vi "DAQ_Main.vi"() -> ()   [LabVIEW 2016]
doc: "Main vi to collect ams data with the pixie 4."
uses:
  spectrum/controls/count control.ctl
  stable current/stable controls/stable cluster.ctl
  record data/realtime data/pixie vis/controls/measurement values.ctl
  record data/realtime data/pixie vis/controls/sample info cluster.ctl
  controls/rare event data.ctl
  controls/stable data.ctl
  controls/main state control.ctl
  controls/SCA broadcast status.ctl
  controls/read write shift control.ctl
  controls/SCA commands.ctl
  <vilib>/addons/database/Connection.llb/DB Tools Open Connec (String).vi
  <vilib>/addons/database/Connection.llb/Conn Execute.vi
  <vilib>/addons/database/Recordset.llb/Rec Fetch Recordset Data (R).vi
  <vilib>/addons/database/Recordset.llb/Rec Destroy - Connection.vi
  <vilib>/Utility/file.llb/Read Delimited Spreadsheet (DBL).vi
  <vilib>/addons/database/NI_Database_API.lvlib
panel:
  out "SCA status":T1
  out "DAQ state control":T2
  in  "Stable Data":T3
  in  "Rare Event Data":T4
  in  "skip sample":bool
  out "Measurement values 3":T5={"Cycle number"=2461.0, "Transmission"=28.91860852171752, "Current 1"=9198.03481365116, " run time"=7.303, "Counts"=606.0, "Live Time"=0.9930715935334873, "Counts per minute"=5013.511490976947, "2nd Current 1"=9198.03481365116, "10Be vs O17"=11.632407319707596, "O17 cycle Error"=52.09583737437704, "rare/stable"=4366.328416433736, "Cycle Error"=1.0, "Interference rate(cps"=144.89870339129973, "total interference counts"=1136.0, "SS Injector "=3.1190766269837584, "SS High End"=2.886696509772986} {"10Be vs O17" format="%#_6f"; "rare/stable" format="%#_6f"}
  in  "use SS ratio":u16(ring) items=["other", "36Cl"]
  out "change sample":i16
  in  "sample change failure":u32(colorbox)
  out "Sample DB fetch error":errorcluster
  in  "2nd sample warm up time 2":dbl=60.0
  in  "Wheel Name":string="tune 1"
  in  "run number":string="201502"
  in  "wheelnumber":string="1"
  in  "runletter":string="2015_14C-01"
  out "run time(sec)":dbl=7.303 format="%#_4g"
  out "sample warm up":u32=200
  in  "number of cycles":u32=4
  in  "1st sample warm up time":dbl=200.0
  in  "run time":dbl=60.0
  out "first time run":bool
  out "recordset data":variant[][](array[variant])
  out "Rare Event Window error":errorcluster
  out "DAQ running SV error":errorcluster
  out "Sample Change Start SV error":errorcluster
  out "input count rate 0":dbl=145.76259366407135
  out "run data output":T6={"input count rate 0"=145.76259366407135, "input count rate 1"=146.1439819888232, "input count rate 2"=0.0, "input count rate 3"=0.0, "number of events"=1136.0, "event rate"=144.89870339129973}
  in  "time for each measurement":i32=500
  in  "data out":T7={"Total counts"=4140, "cps"=80.49411774042008, "live time"=0.9916920520631404, "pulser"=3611.0, "rare counts"=4809.0, "other counts"=4294958918.0, "total run time(sec)"=60.244, "adjusted run time(sec)"=59.74349598449183, "17O average"=4.140581045750721, "17O current"=372.65229411756485}
  in  "abort count rate (cps)":dbl=40000.0
  in  "reset":bool
  out "rare count rate":dbl=54.0 format="%#_3g"
  out "DB input error":errorcluster
  in  "13 to 12 conversion .011 for 14C otherwise 1":dbl=1.0
  in  "Charge State":dbl=3.0
  out "Measurement values 2":T8={"Cycle number"=2461.0, "Transmission"=28.91860852171752, "Current 1"=9198.03481365116, " run time"=7.303, "Counts"=606.0, "Live Time"=0.9930715935334873, "Counts per minute"=5013.511490976947, "2nd Current 1"=9198.03481365116, "10Be vs O17"=11.632407319707596, "O17 cycle Error"=52.09583737437704, "rare/stable"=4366.328416433736, "Cycle Error"=1.0, "Interference rate(cps"=144.89870339129973, "total interference counts"=1136.0, "SS Injector "=3.1190766269837584, "SS High End"=2.886696509772986} {"10Be vs O17" format="%#_6f"; "rare/stable" format="%#_6f"}
  out "Sample information":T9={"Cathode Number"="124120", "Sample Name"="26Al-01-5-1", "Type"="s", "User Name"="Caffee", "Cycles Measured"="1", "Cathode Position"="10", "Estimated Ratio"="4694"}
  in  "Measurement values":T8={"Cycle number"=2460.0, "Transmission"=24.878524366136492, "Current 1"=7973.094300785374, " run time"=60.244, "Counts"=4809.0, "Live Time"=0.9916920520631404, "Counts per minute"=4829.647064425205, "2nd Current 1"=7951.125552694256, "10Be vs O17"=12.904791077128992, "O17 cycle Error"=372.65229411756485, "rare/stable"=4859.10919175385, "Cycle Error"=1.0, "Interference rate(cps"=140.58271554902092, "total interference counts"=8495.0, "SS Injector "=3.1190766269837584, "SS High End"=2.886696509772986} {"10Be vs O17" format="%#_6f"; "rare/stable" format="%#_6f"}
  out "millisecond timer value":u32
  out "Wheel run order array":string[][](array[string])=[["10", "124120", "Caffee", "26Al-01-5-1", "s", "4694", "0", "Finished"], ["13", "109265", "Caffee", "QA-Al-16760", "u", "16760", "0", ""], ["12", "124831", "Caffee", "QA-Al-10650", "u", "10650", "0", ""], ["11", "123809", "Caffee", "QA-Al-499", "u", "499", "0", ""], ["4", "124041", "Sharma", "Blank", "b", "5", "0", ""], ["9", "124119", "Caffee", "26Al-01-5-1", "s", "4694", "0", ""], ["3", "124039", "Sharma", "Blank", "b", "5", "0", ""], ["2", "124035", "Sharma", "Blank", "b", "5", "0", ""], ["1", "124031", "Sharma", "Blank", "b", "5", "0", ""], ["8", "124118", "Caffee", "26Al-01-5-1", "s", "4694", "0", ""], ["10", "124120", "Caffee", "26Al-01-5-1", "s", "4694", "0", ""], ["13", "109265", "Caffee", "QA-Al-16760", "u", "16760", "0", ""], ["12", "124831", "Caffee", "QA-Al-10650", "u", "10650", "0", ""], ["11", "123809", "Caffee", "QA-Al-499", "u", "499", "0", ""], ["4", "124041", "Sharma", "Blank", "b", "5", "0", ""], ["9", "124119", "Caffee", "26Al-01-5-1", "s", "4694", "0", ""], ["3", "124039", "Sharma", "Blank", "b", "5", "0", ""], ["2", "124035", "Sharma", "Blank", "b", "5", "0", ""], ["1", "124031", "Sharma", "Blank", "b", "5", "0", ""], ["8", "124118", "Caffee", "26Al-01-5-1", "s", "4694", "0", ""], ["10", "124120", "Caffee", "26Al-01-5-1", "s", "4694", "0", ""], ["13", "109265", "Caffee", "QA-Al-16760", "u", "16760", "0", ""], ["12", "124831", "Caffee", "QA-Al-10650", "u", "10650", "0", ""], ["11", "123809", "Caffee", "QA-Al-499", "u", "499", "0", ""], ["4", "124041", "Sharma", "Blank", "b", "5", "0", ""], ["9", "124119", "Caffee", "26Al-01-5-1", "s", "4694", "0", ""], ["3", "124039", "Sharma", "Blank", "b", "5", "0", ""], ["2", "124035", "Sharma", "Blank", "b", "5", "0", ""], ["1", "124031", "Sharma", "Blank", "b", "5", "0", ""], ["8", "124118", "Caffee", "26Al-01-5-1", "s", "4694", "0", ""]]
  out "sample number":u16=57
  in  "stable data out 2":T10={"injector current"=10618.359999999999, "offset current"=7973.094300785374, "ss inj ratio"=3.1190766269837584, "ss offset ratio"=2.886696509772986, "transmission"=25.029271001000076, "2nd offset current"=7951.125552694256}
  out "stable data out":T10={"injector current"=10602.21, "offset current"=9198.03481365116, "ss inj ratio"=3.1190766269837584, "ss offset ratio"=2.886696509772986, "transmission"=28.91860852171752, "2nd offset current"=9198.03481365116}
  out "data":T7={"Total counts"=962, "cps"=83.5585248496158, "live time"=0.9930715935334873, "pulser"=433.0, "rare counts"=606.0, "other counts"=4294966311.0, "total run time(sec)"=7.303, "adjusted run time(sec)"=7.252401847575058, "17O average"=4.735985215852458, "17O current"=52.09583737437704}
  out "Event structure error out":errorcluster
  in  "run":bool=TRUE
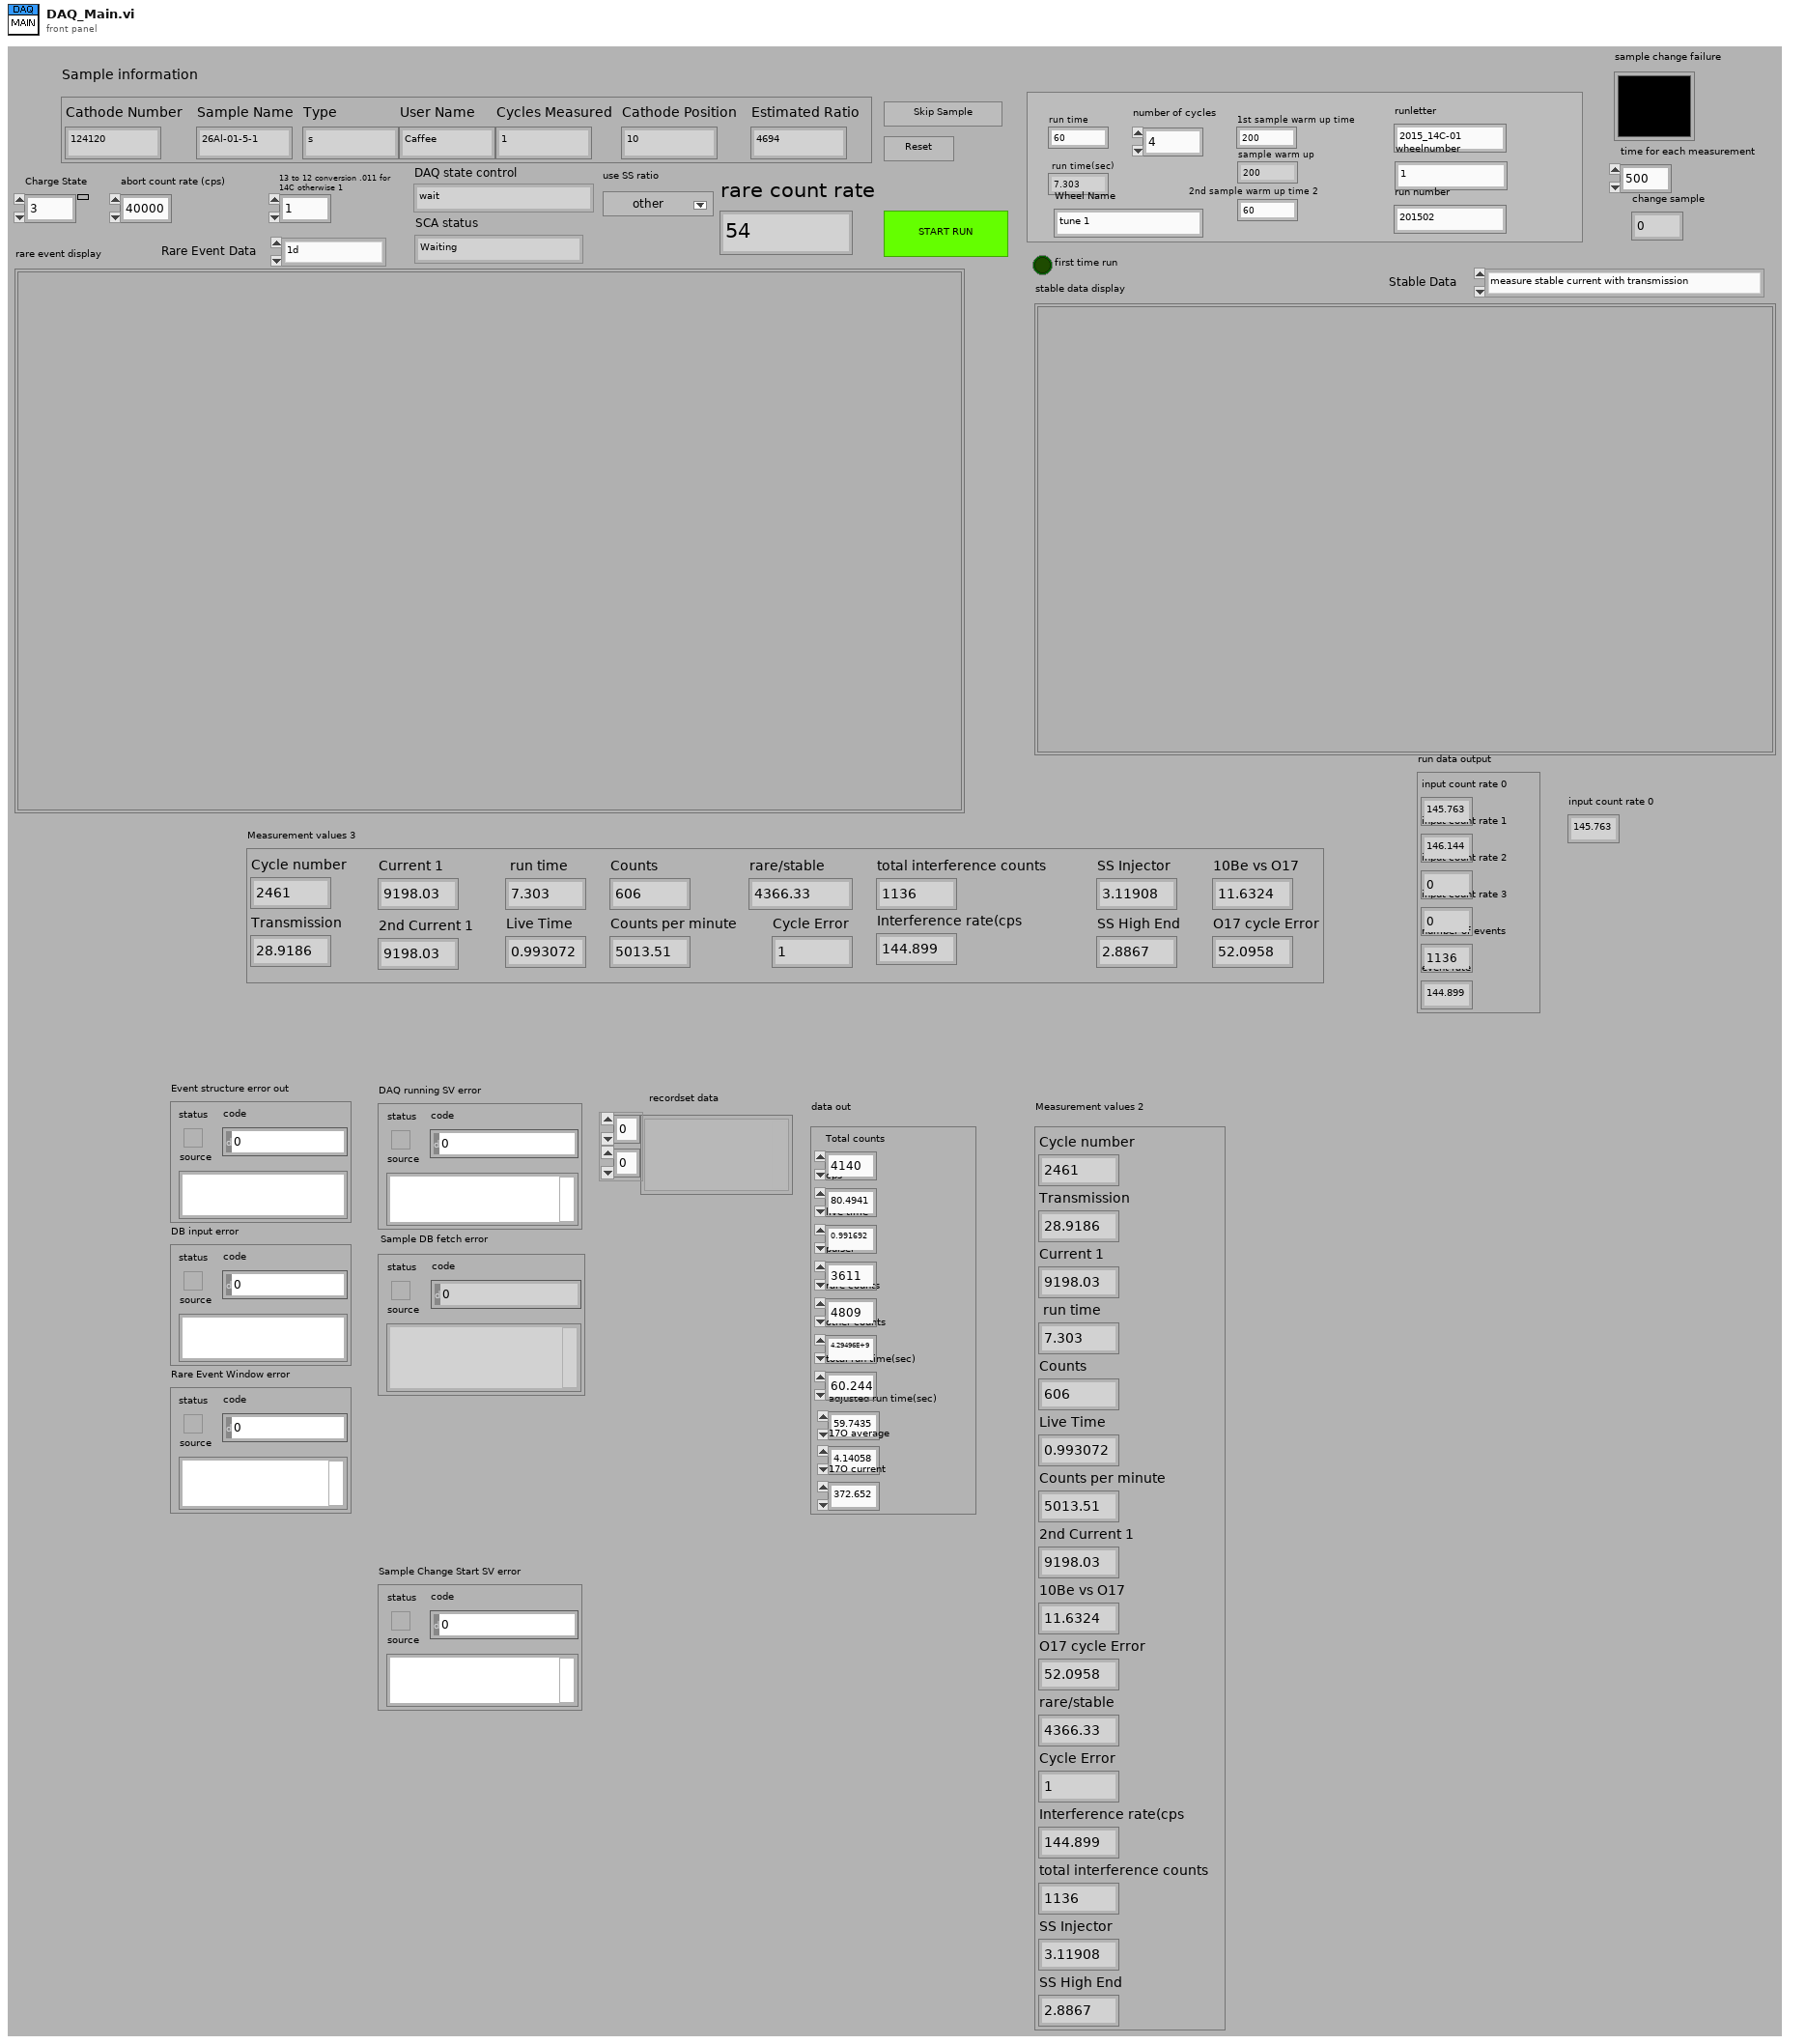
[diagram p1: front panel]
types:
  T1 = typedef "SCA broadcast status.ctl" = enum16{"Waiting", "Changing samples", "Sample change complete", "Failure"}
  T2 = typedef "main state control.ctl" = enum16{"wait", "set gate", "check injector cup", "start rare", "get rare", "stop rare", "abort run", "change sample", "wait for sample change", "check sample start", "insert cup", "remove cup", "sample warm up", "record data", "get transmission", "get stable"}
  T3 = typedef "stable data.ctl" = enum16{"measure stable current with transmission", "measure stable current", "35Cl + 37Cl measure stable current", "35Cl + 37Cl inj - 35Cl HE"}
  T4 = typedef "rare event data.ctl" = enum16{"1d", "2d", "2d 10Be"}
  T5 = cluster{"Cycle number":dbl, "Transmission":dbl, "Current 1":dbl, " run time":dbl, "Counts":dbl, "Live Time":dbl, "Counts per minute":dbl, "2nd Current 1":dbl, "10Be vs O17":dbl, "O17 cycle Error":dbl, "rare/stable":dbl, "Cycle Error":dbl, "Interference rate(cps":dbl, "total interference counts":dbl, "SS Injector ":dbl, "SS High End":dbl}
  T6 = cluster{"input count rate 0":dbl, "input count rate 1":dbl, "input count rate 2":dbl, "input count rate 3":dbl, "number of events":dbl, "event rate":dbl}
  T7 = typedef "count control.ctl" = cluster{"Total counts":u32, "cps":dbl, "live time":dbl, "pulser":dbl, "rare counts":dbl, "other counts":dbl, "total run time(sec)":dbl, "adjusted run time(sec)":dbl, "17O average":dbl, "17O current":dbl}
  T8 = typedef "measurement values.ctl" = cluster{"Cycle number":dbl, "Transmission":dbl, "Current 1":dbl, " run time":dbl, "Counts":dbl, "Live Time":dbl, "Counts per minute":dbl, "2nd Current 1":dbl, "10Be vs O17":dbl, "O17 cycle Error":dbl, "rare/stable":dbl, "Cycle Error":dbl, "Interference rate(cps":dbl, "total interference counts":dbl, "SS Injector ":dbl, "SS High End":dbl}
  T9 = typedef "sample info cluster.ctl" = cluster{"Cathode Number":string, "Sample Name":string, "Type":string, "User Name":string, "Cycles Measured":string, "Cathode Position":string, "Estimated Ratio":string}
  T10 = typedef "stable cluster.ctl" = cluster{"injector current":dbl, "offset current":dbl, "ss inj ratio":dbl, "ss offset ratio":dbl, "transmission":dbl, "2nd offset current":dbl}
  T11 = cluster{"array out[0]":string, "array out[1]":string, "array out[2]":string, "array out[3]":string, "array out[4]":string, "array out[5]":string, "array out[6]":string}
  T12 = typedef "read write shift control.ctl" = string
  T13 = typedef "SCA commands.ctl" = enum16{"Wait", "Shutdown", "Retract insert rod", "Insert insert rod", "Retract retract rod", "Insert retract rod", "Retract sample rod", "Insert sample rod", "Open wheel GV", "Close wheel GV", "Open ion source GV", "Close ion source GV", "Pump out source", "Vent source", "Rotate wheel randomly", "Rotate wheel", "Start random sample change", "Start sample change"}
  T14 = enum16{"open", "replace", "create", "open or create", "replace or create", "replace or create with confirmation"}
  T15 = typedef "NI_Database_API.lvlib/Conn ObjectReference.ctl" = refnum<k1>
  T16 = typedef "NI_Database_API.lvlib/Rec ObjectReference.ctl" = refnum<k1>
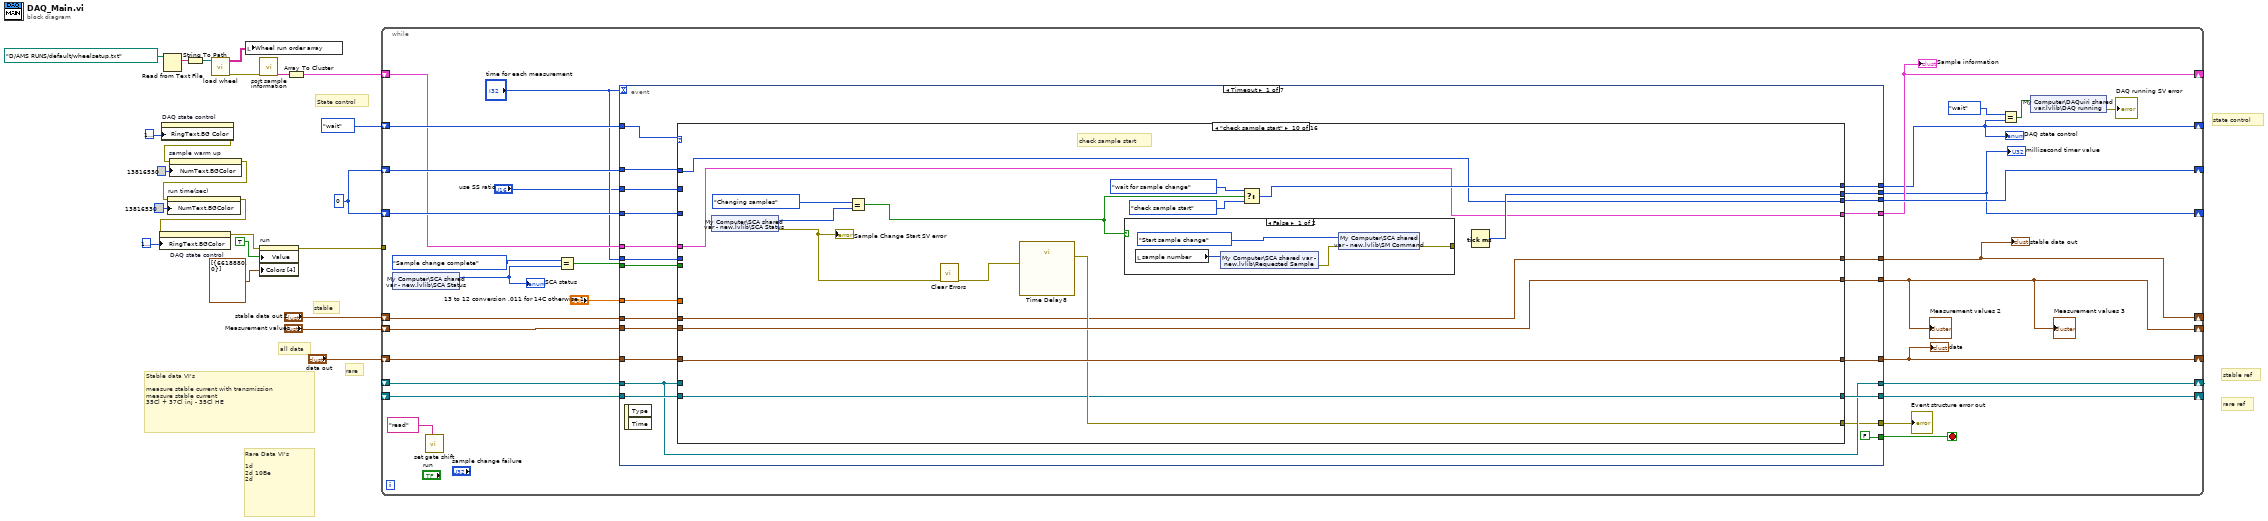
[diagram p0: block diagram]
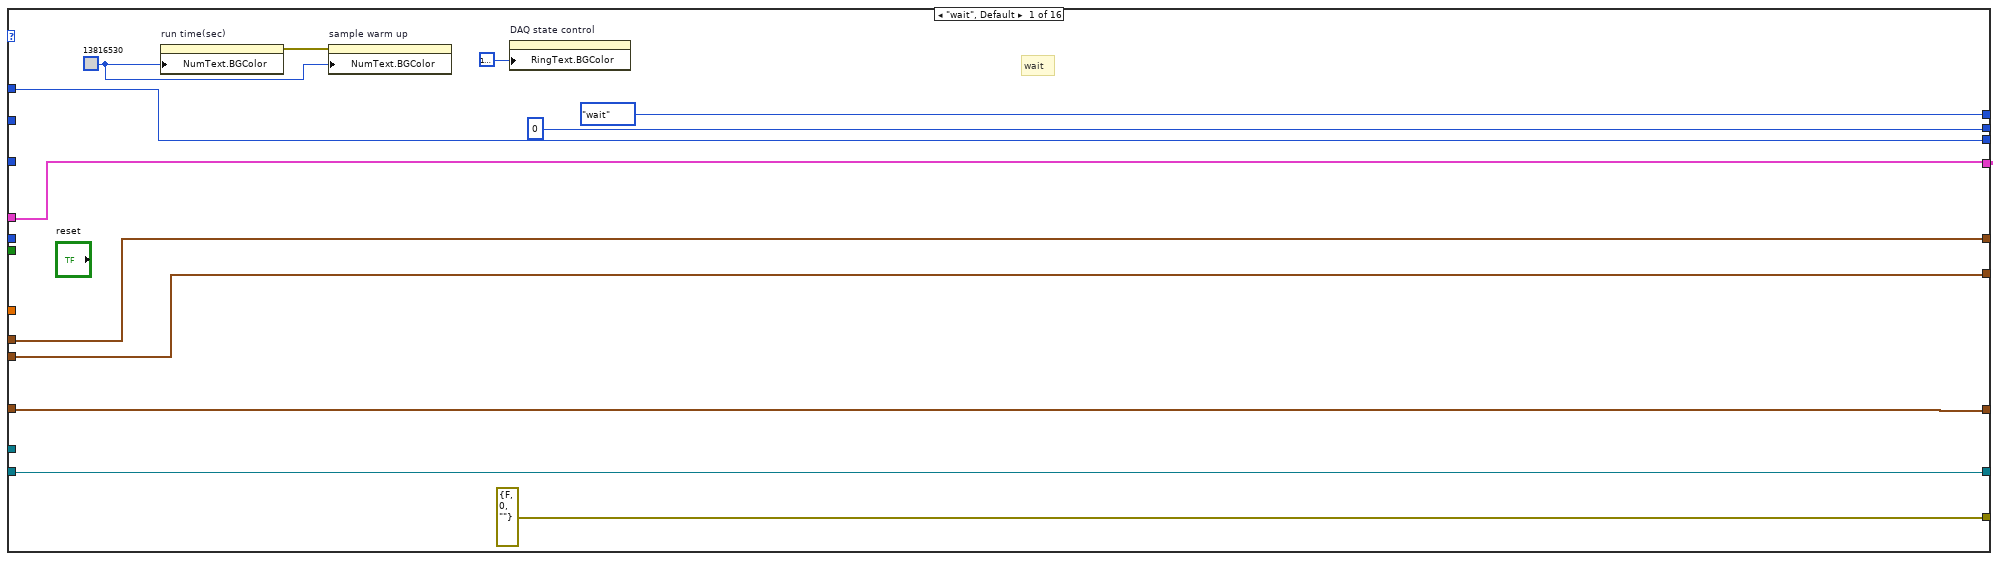
[diagram p2: hidden frame]
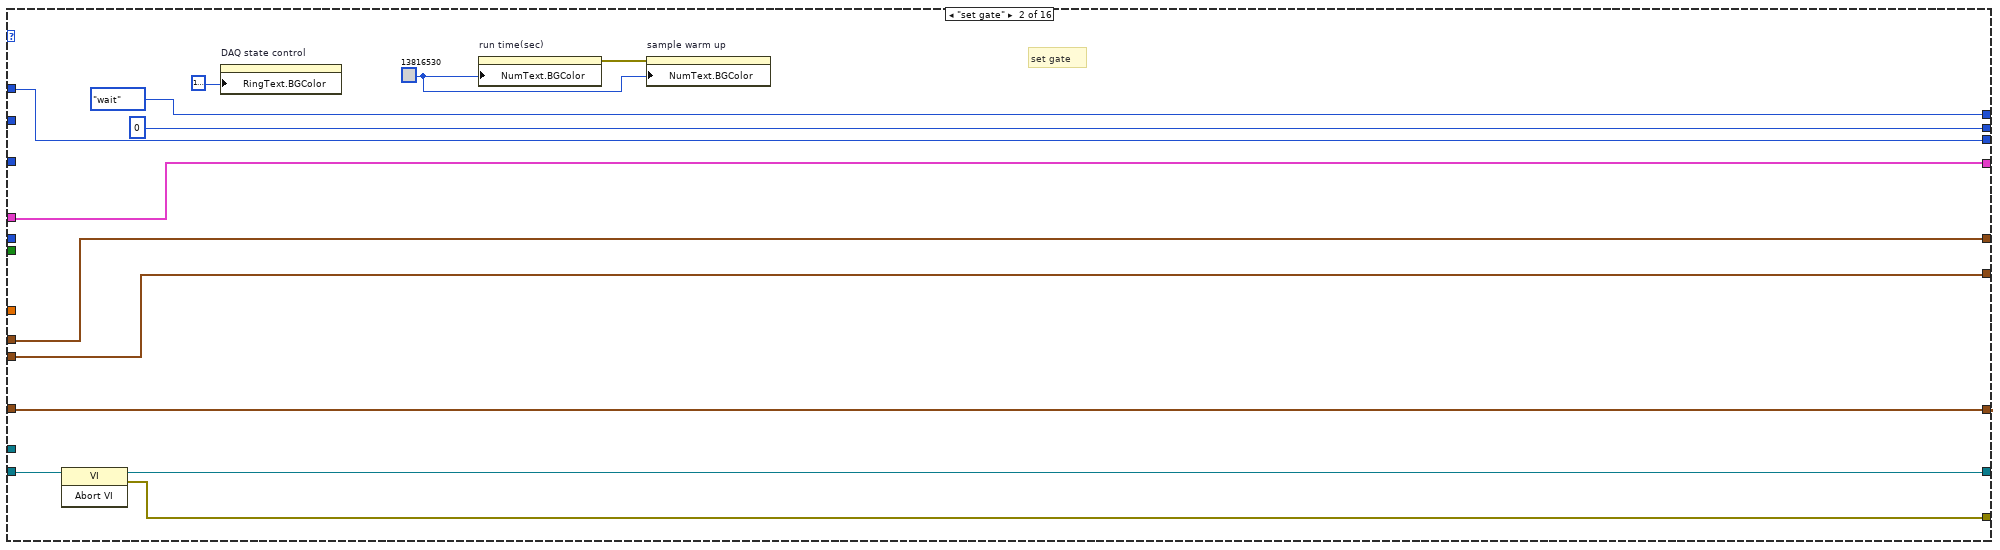
[diagram p3: hidden frame]
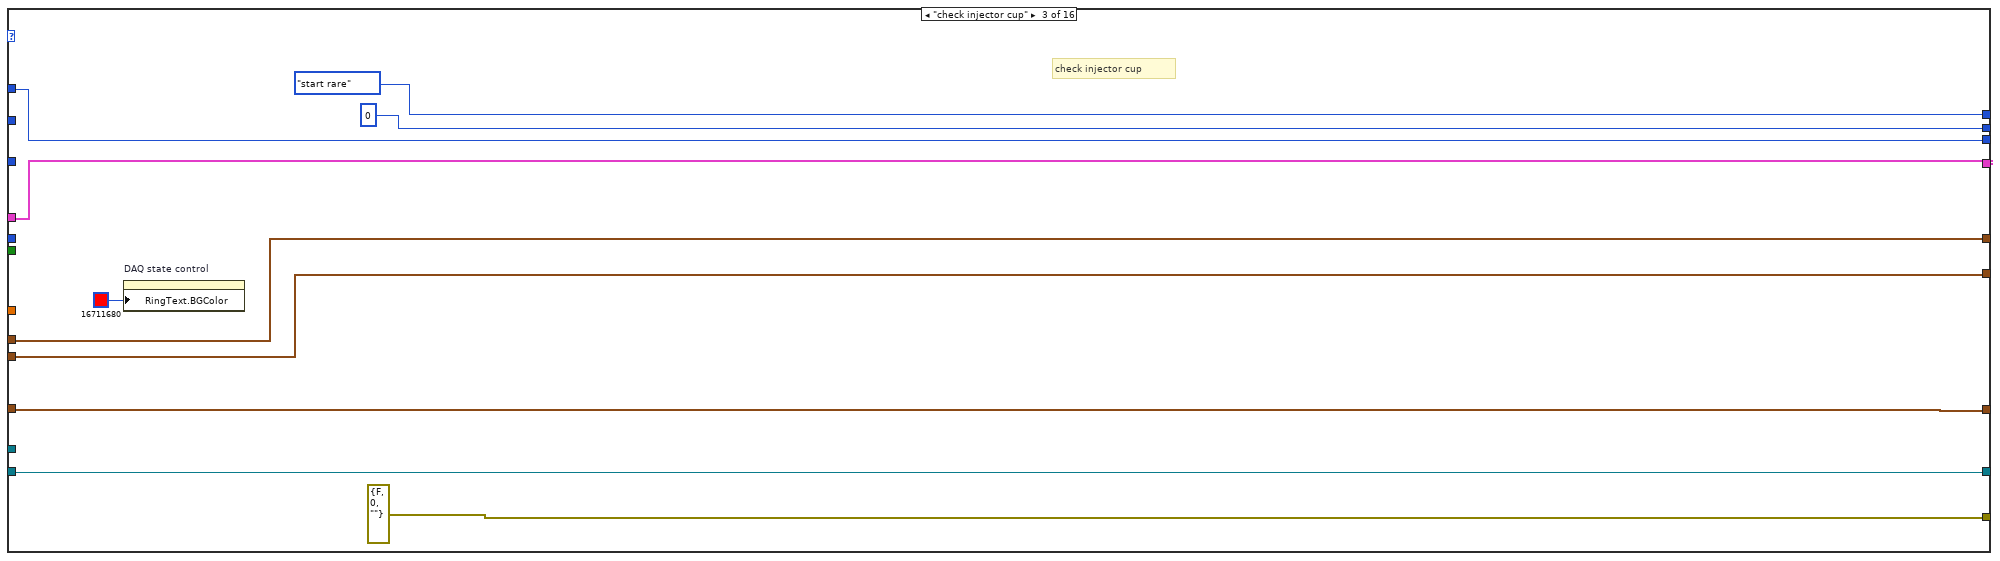
[diagram p4: hidden frame]
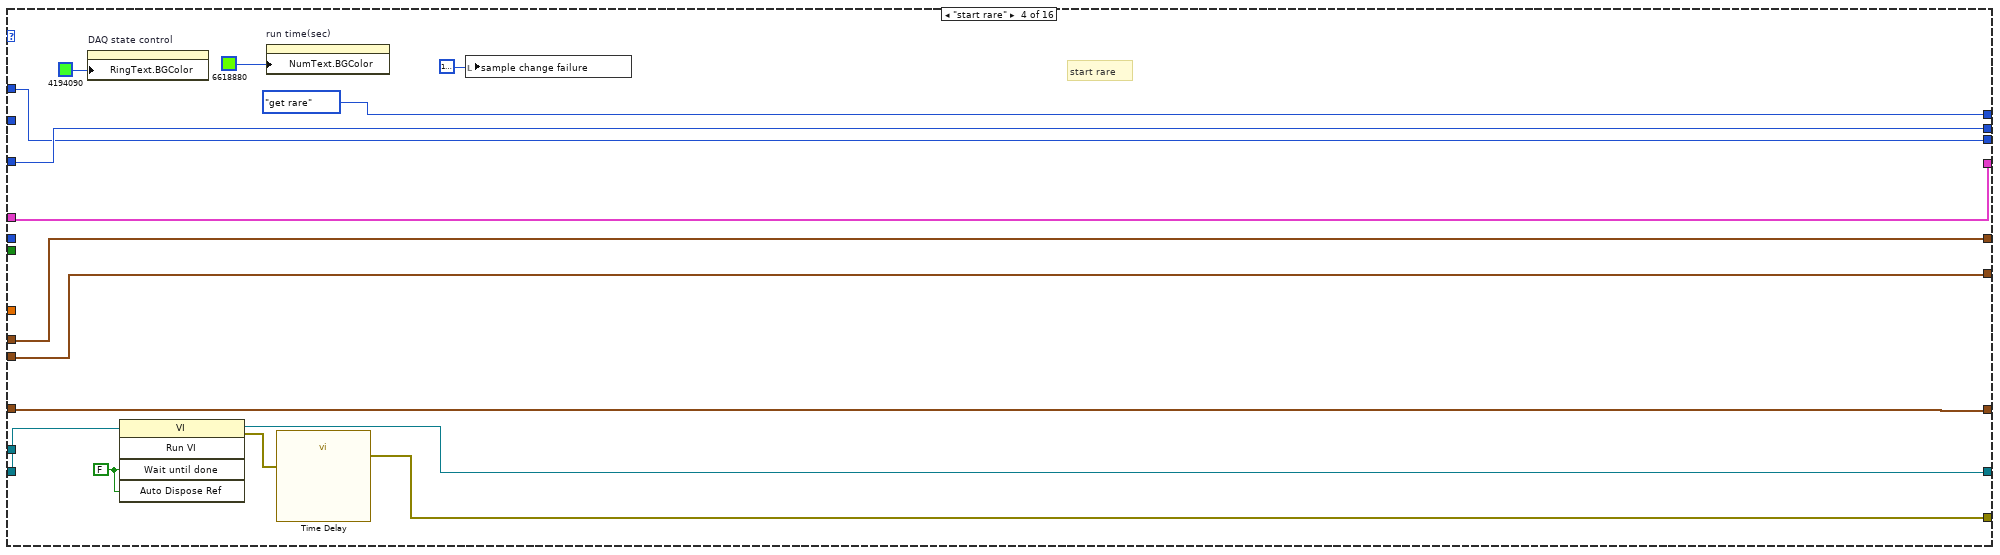
[diagram p5: hidden frame]
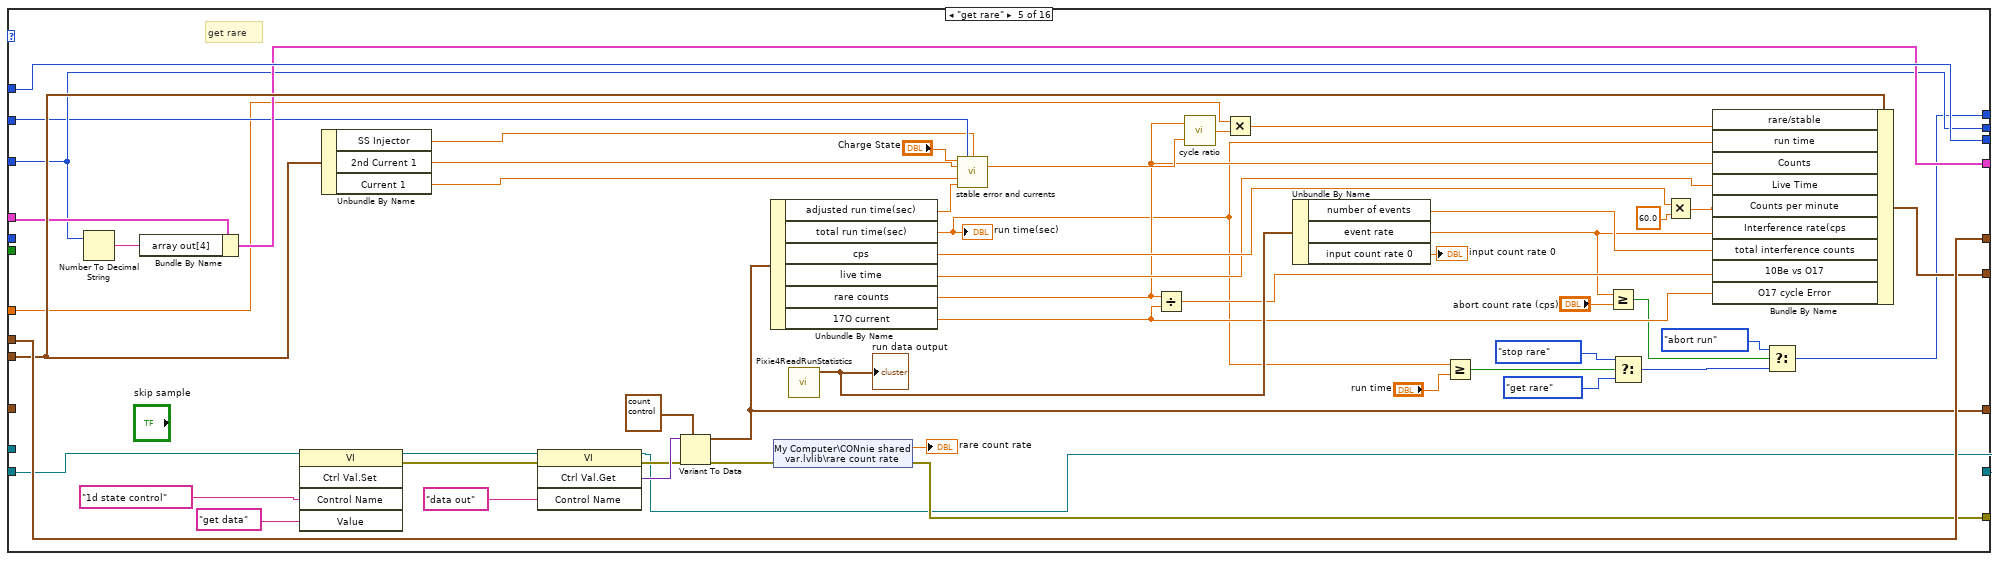
[diagram p6: hidden frame]
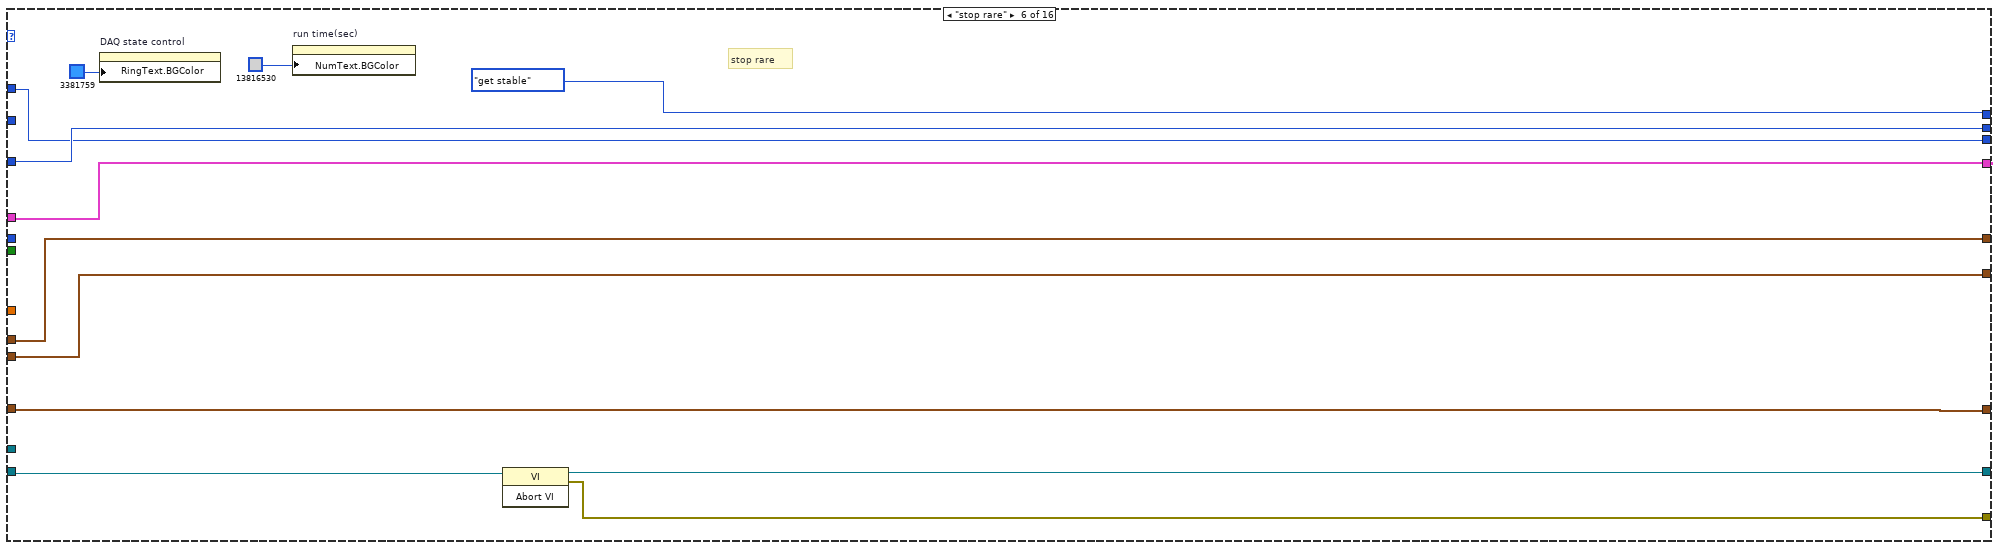
[diagram p7: hidden frame]
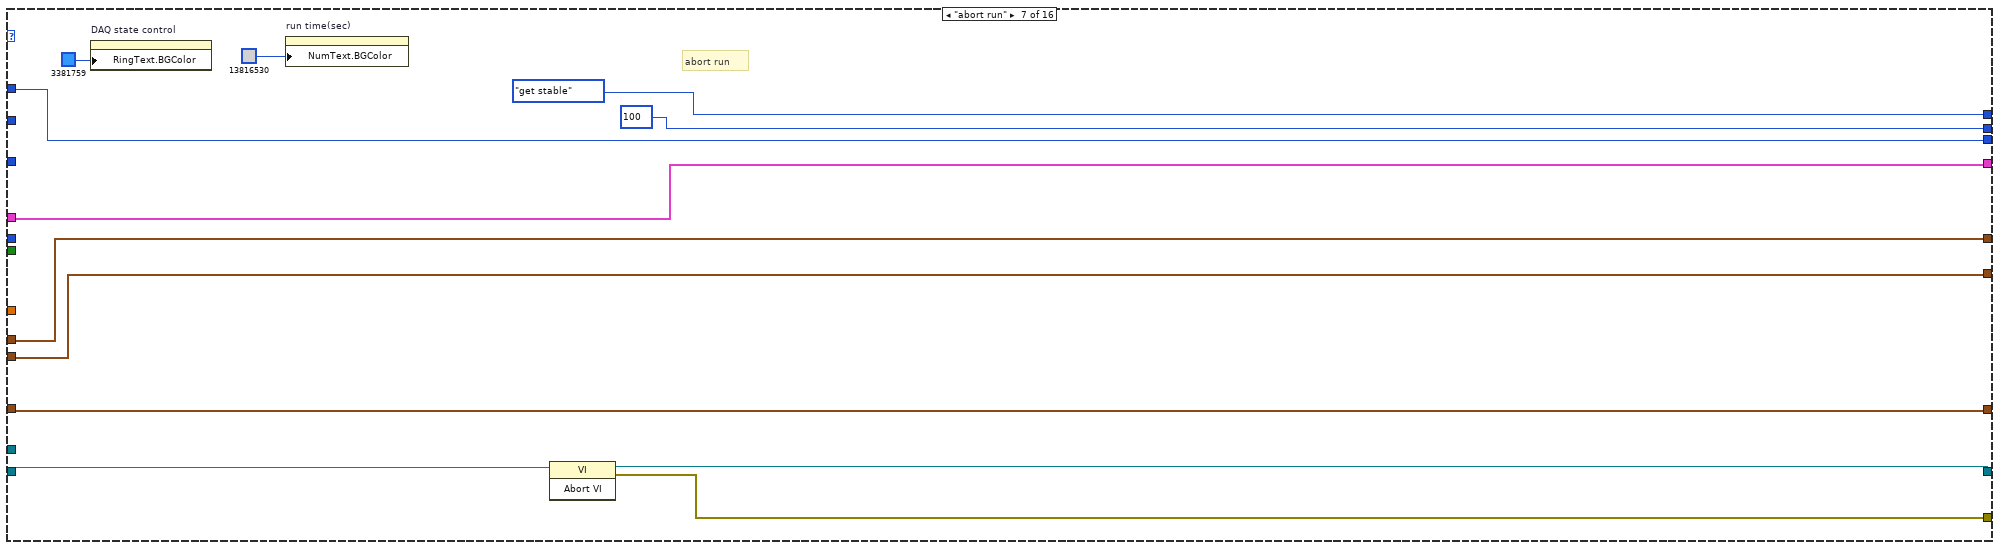
[diagram p8: hidden frame]
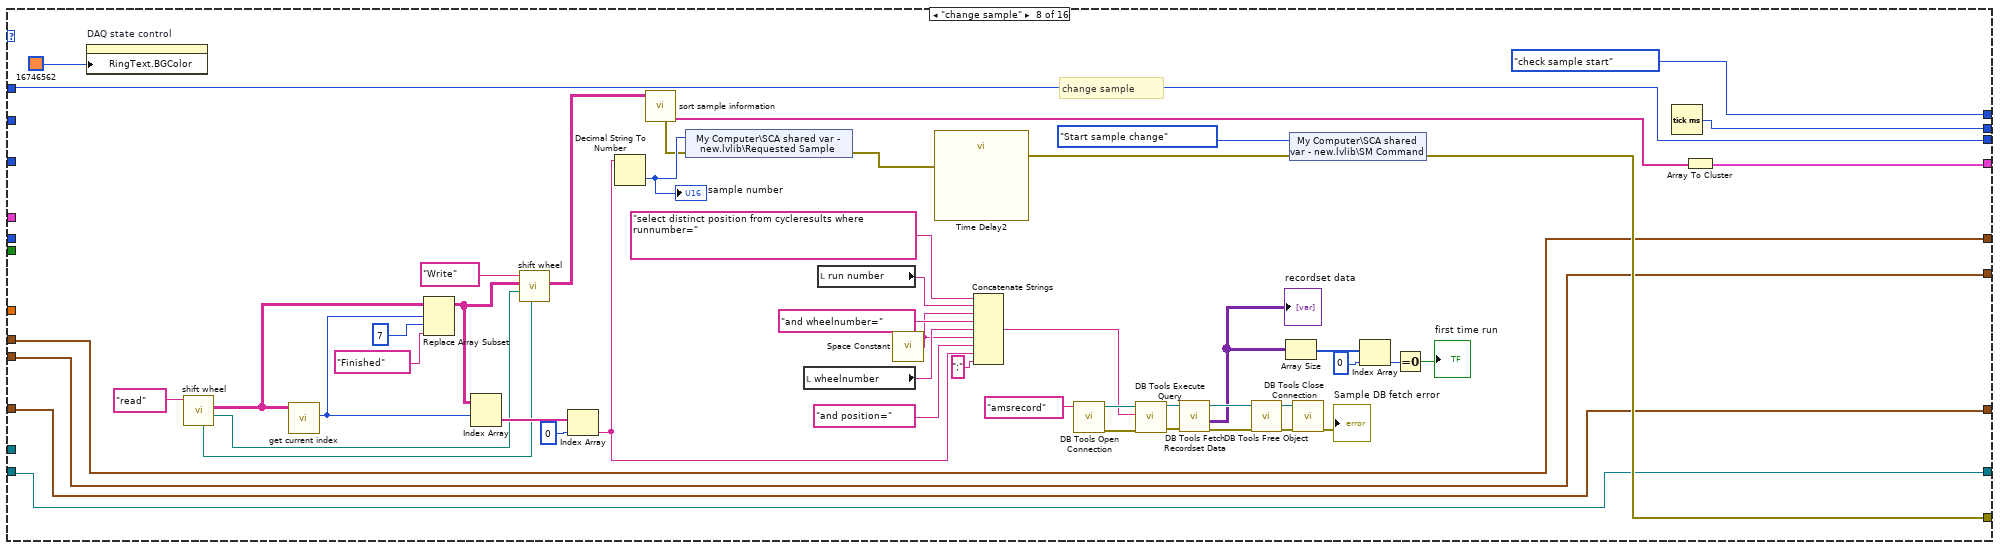
[diagram p9: hidden frame]
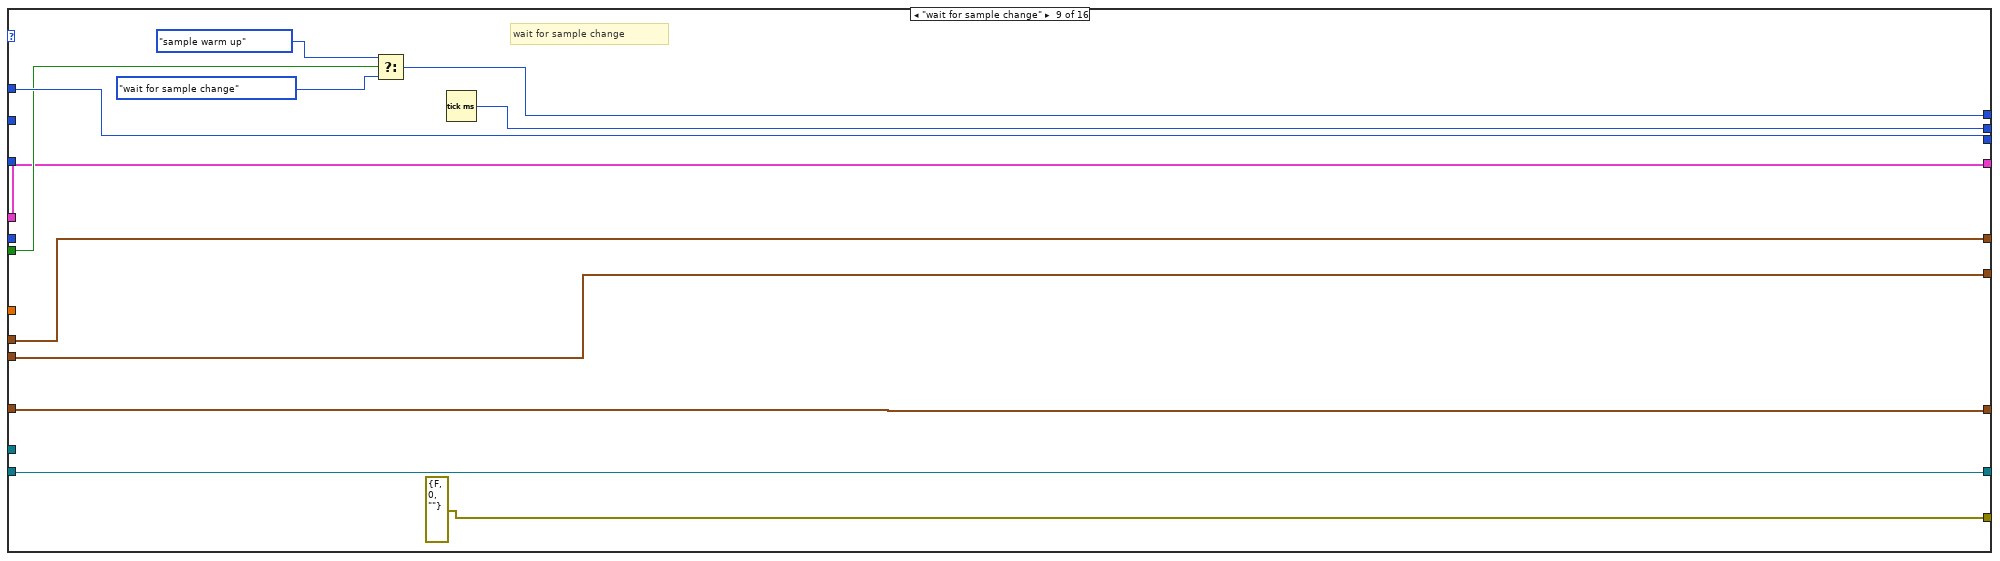
[diagram p10: hidden frame]
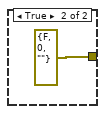
[diagram p11: hidden frame]
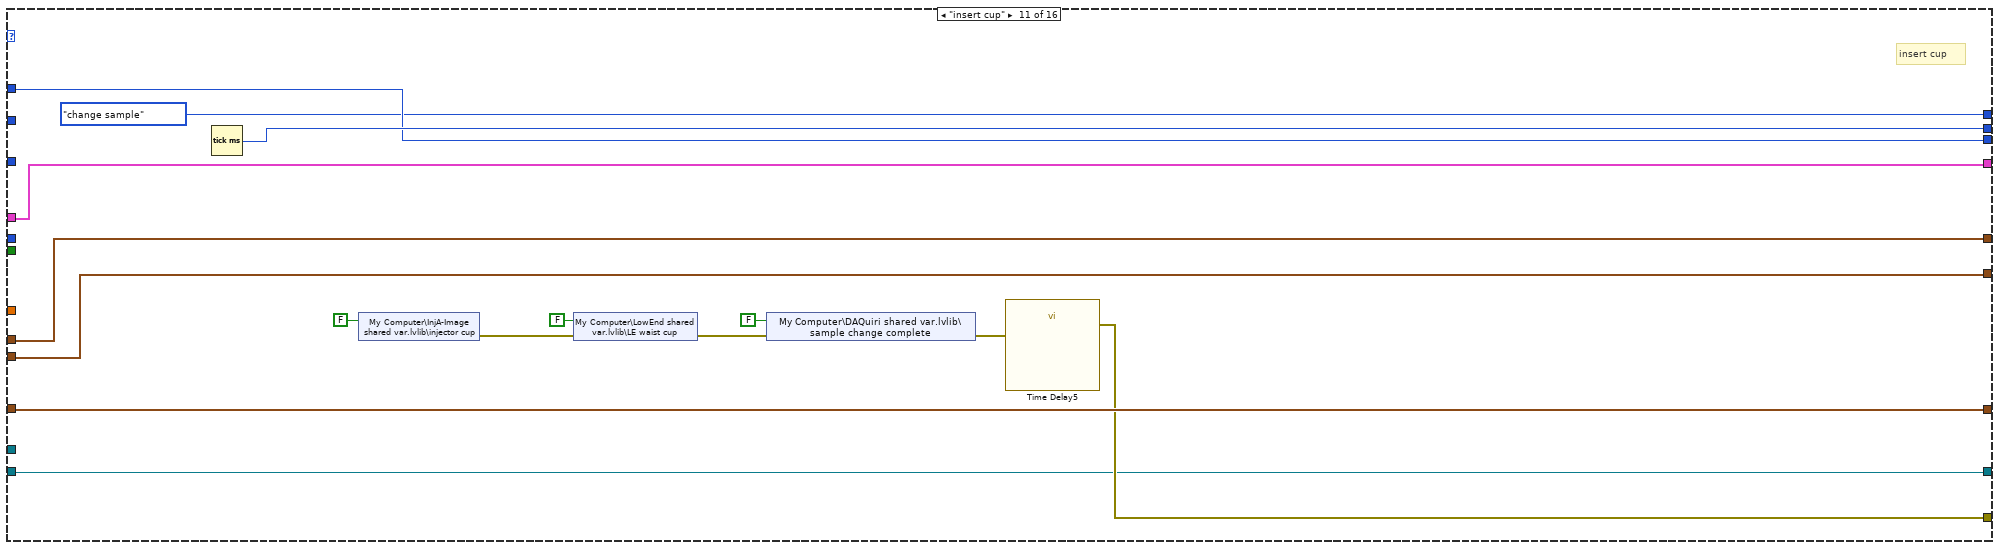
[diagram p12: hidden frame]
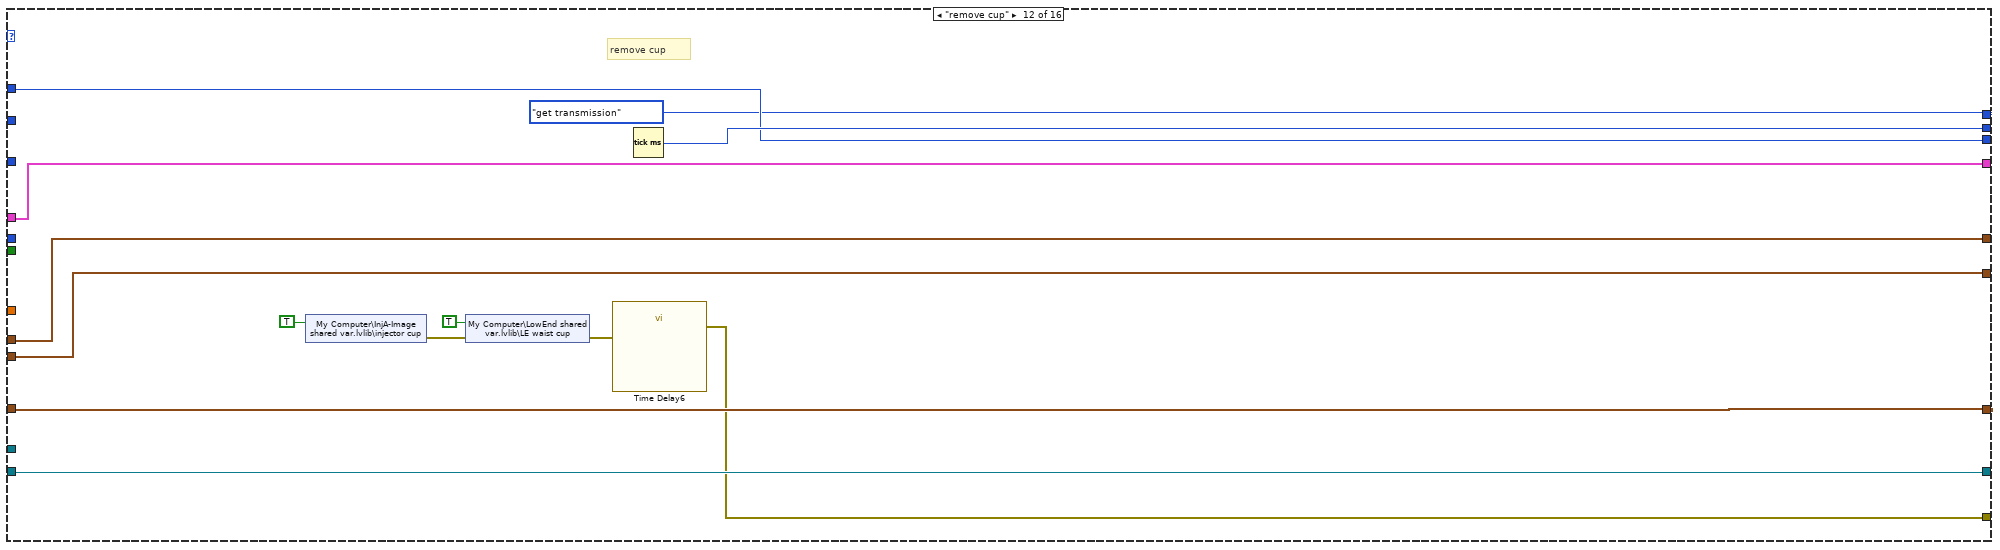
[diagram p13: hidden frame]
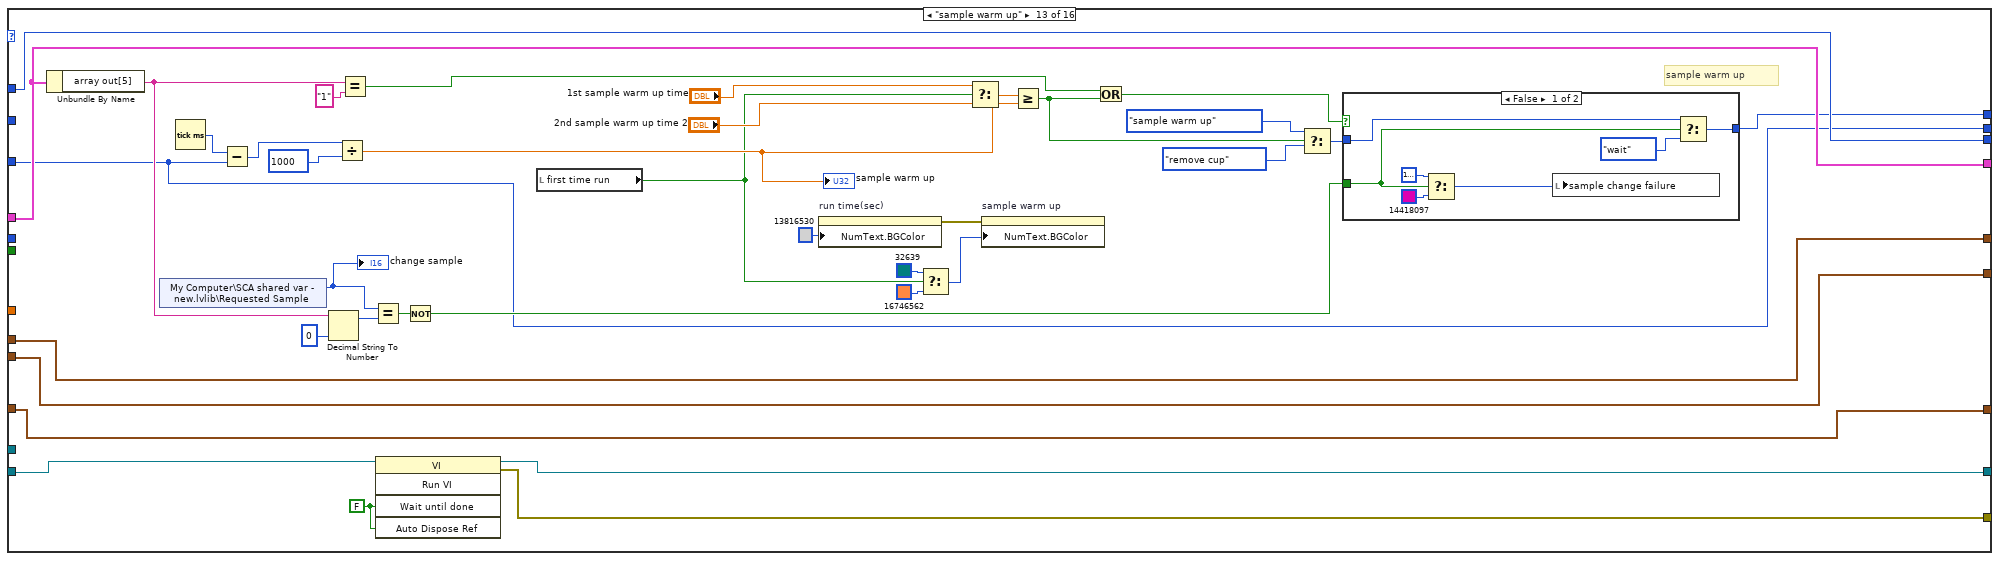
[diagram p14: hidden frame]
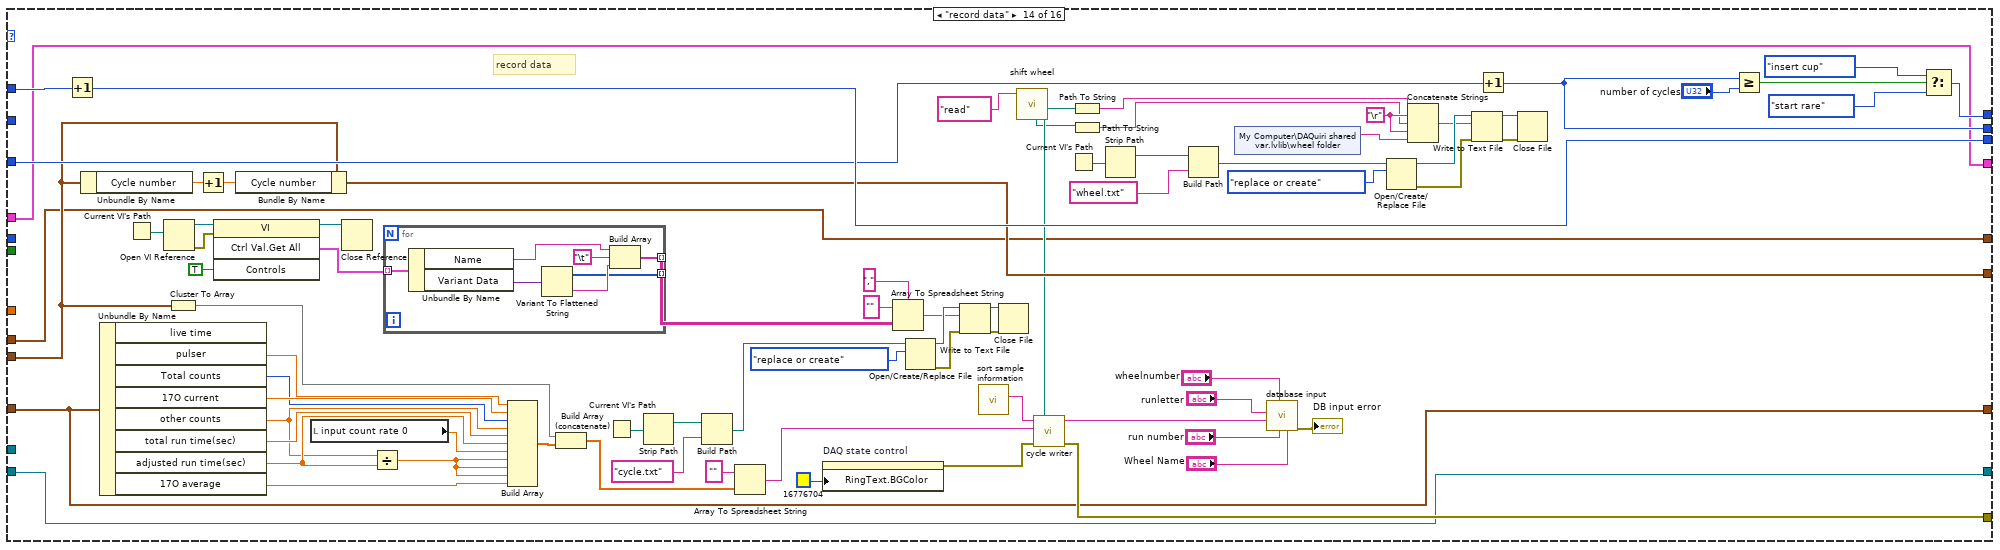
[diagram p16: hidden frame]
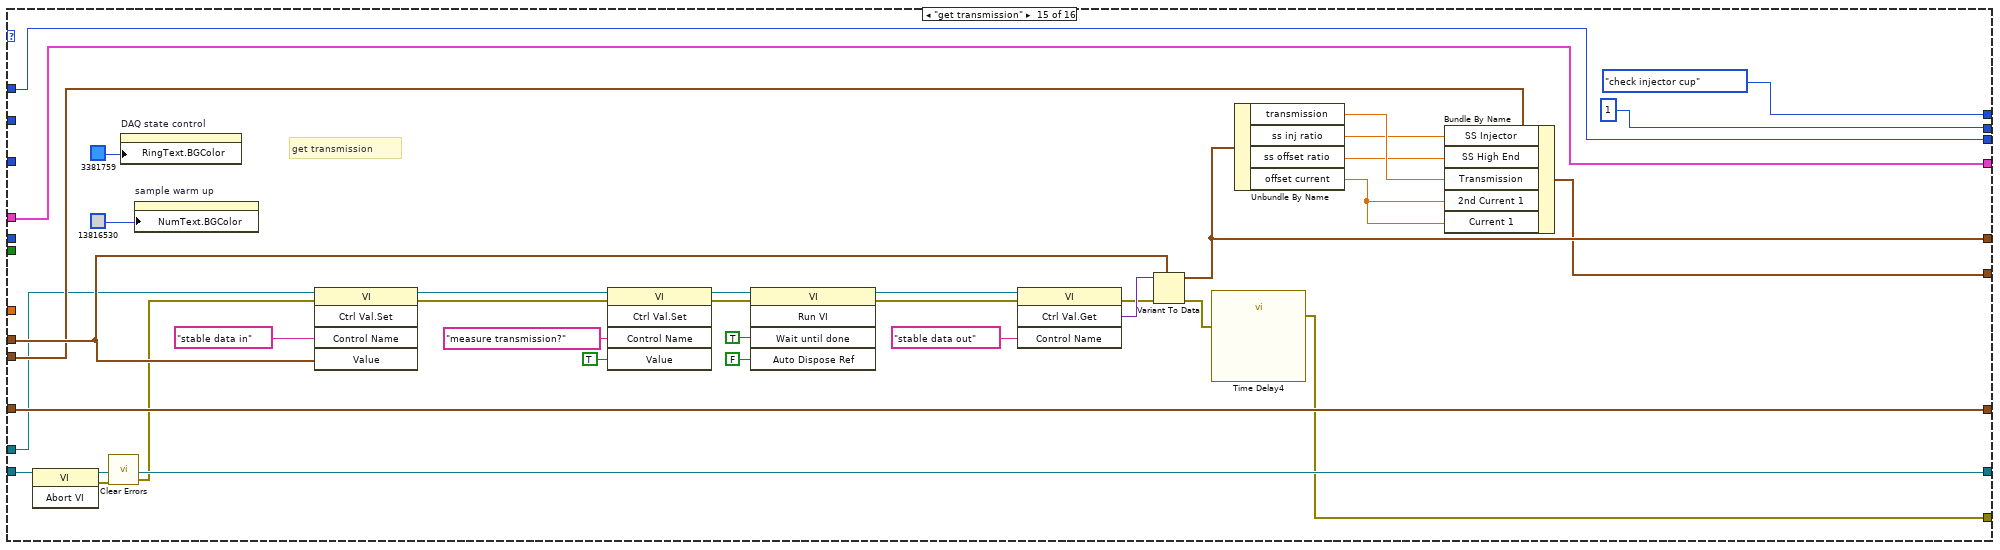
[diagram p17: hidden frame]
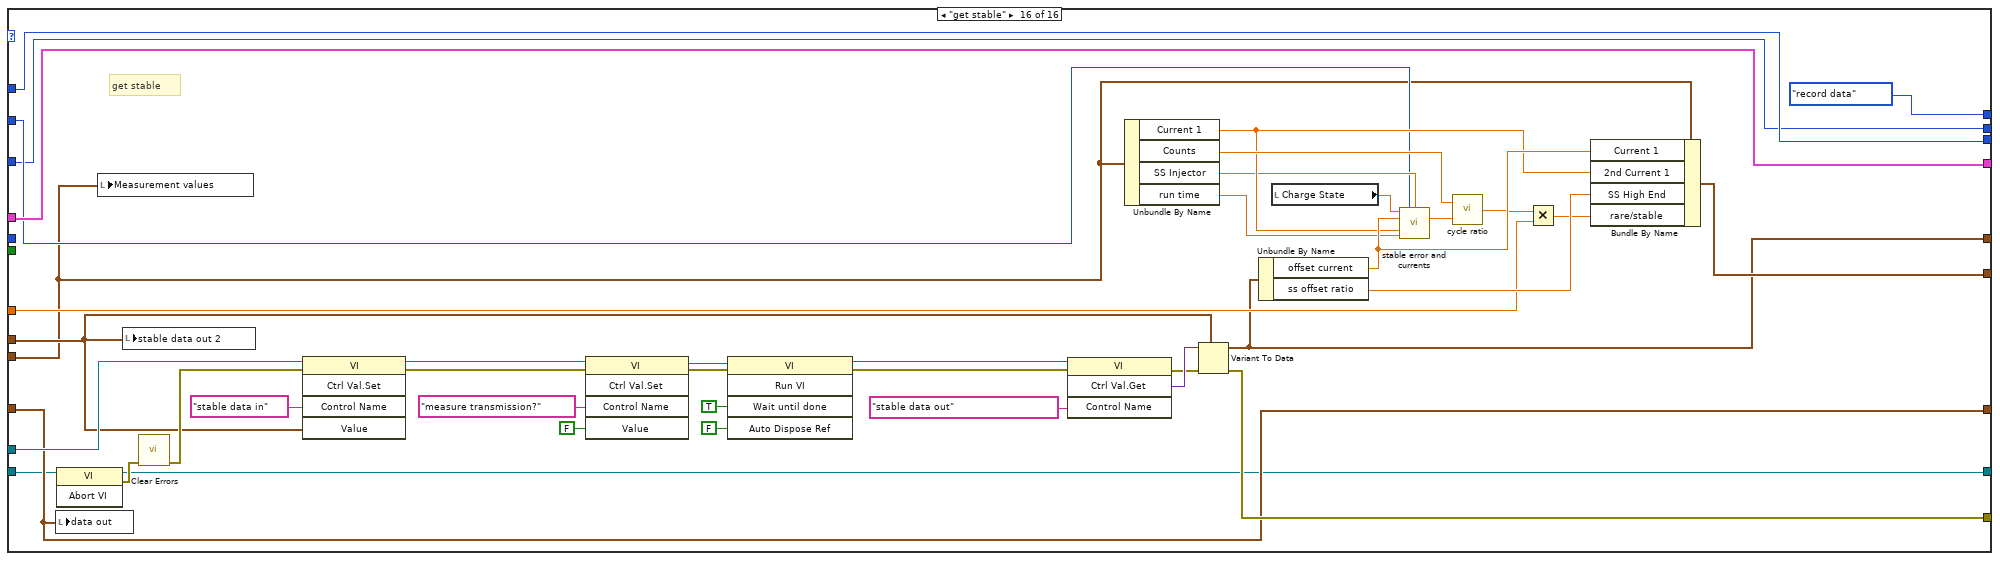
[diagram p18: hidden frame]
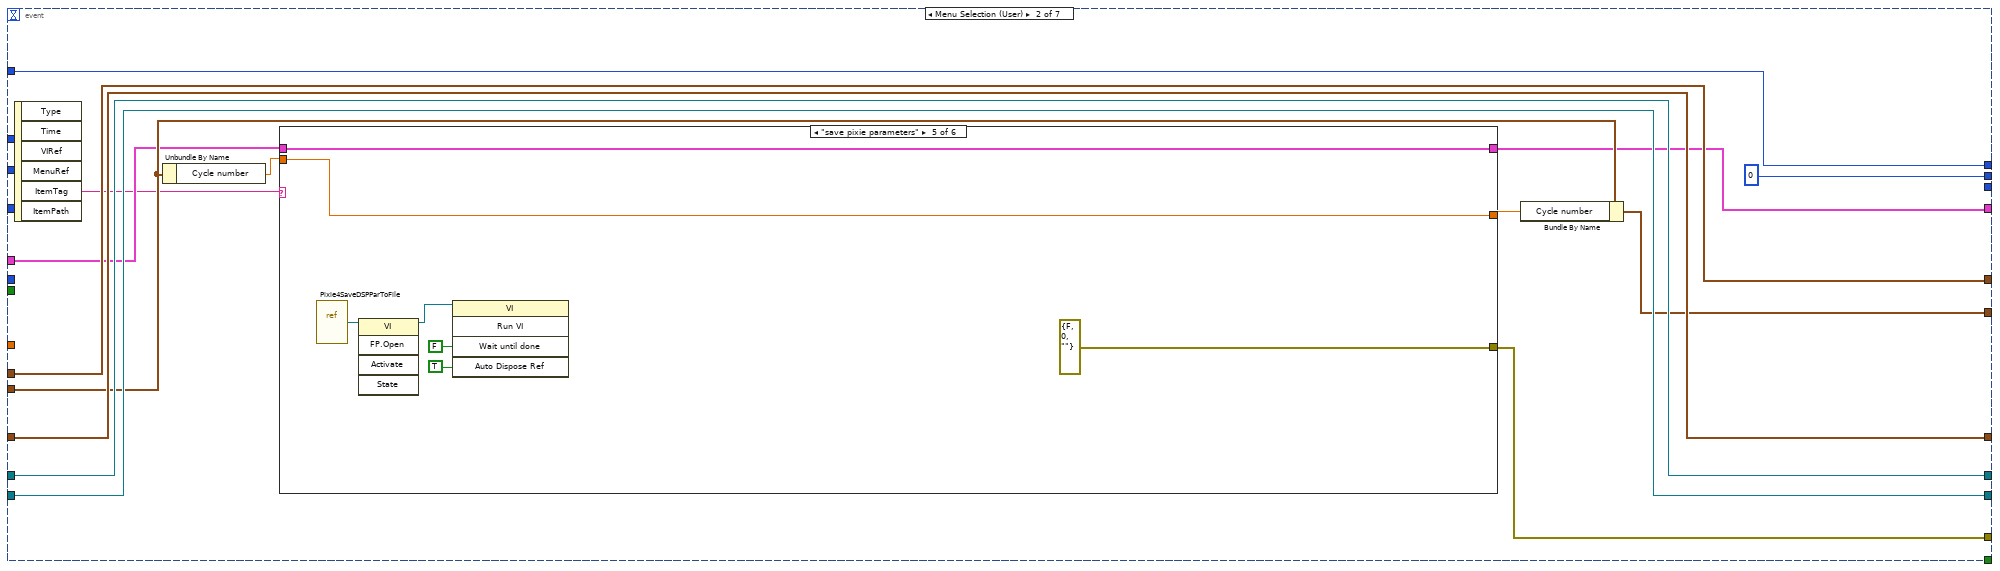
[diagram p19: hidden frame]
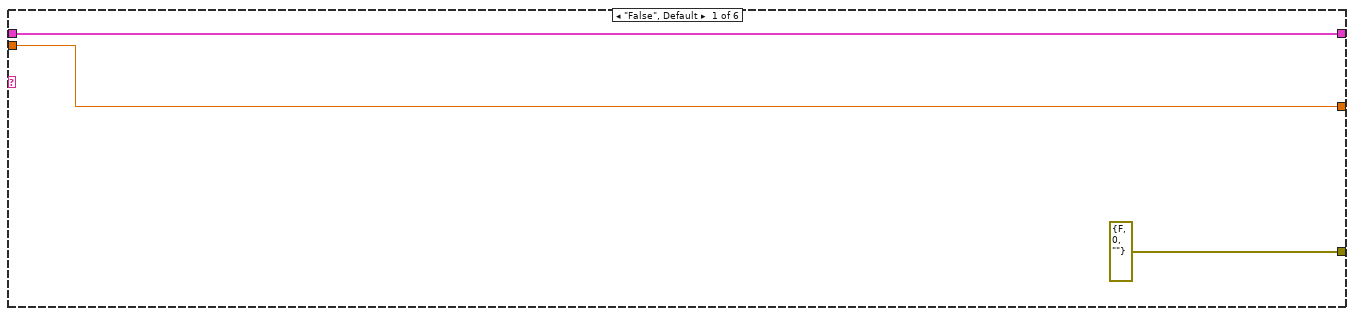
[diagram p20: hidden frame]
diagram:
  w22 = u32 0 ("millisecond timer value")
  # "rare"
  # "stable"
  # "all data"
  # "State control"
  # "stable ref"
  # "state control"
  # "rare ref"
  # "Rare Data VI's\n\n1d\n2d 10Be\n2d"
  # "Stable data VI's\n\nmeasure stable current with transmission\nmeasure stable current\n35Cl + 37Cl inj - 35Cl HE"
  n1 = property on="DAQ state control" class="Enum (strict)"("RingText.BG Color"=u32 16777238) -> (error out=w4:errorcluster)  [unwired: 2 in, 1 out]
  n2 = Read from Text File(file (use dialog)=path "D:/AMS RUNS/default/wheelsetup.txt") -> (text=w10:string)  [unwired: 3 in, 3 out]
  n3 = property on="sample warm up" class="DigNum (strict)"(error in=w4, "NumText.BGColor"=u32 13816530) -> (error out=w3:errorcluster)  [unwired: 1 in, 1 out]
  n4 = property on="run time(sec)" class="DigNum (strict)"(error in=w3, "NumText.BGColor"=u32 13816530) -> (error out=w2:errorcluster)  [unwired: 1 in, 1 out]
  n5 = property on="DAQ state control" class="Enum (strict)"(error in=w2, "RingText.BGColor"=u32 16777238) -> (error out=w6:errorcluster)  [unwired: 1 in, 1 out]
  n6 = String To Path(string=w10) -> (path=w9:path)
  n7 = call "load wheel.vi"("file path"=w9) -> ("error out"=w12:errorcluster, "Wheel run order array"=w13:string[][])  [unwired: 7 in, 2 out]
  n8 = local write "Wheel run order array"(w13) -> ()
  n9 = call "sort sample information.vi"("error in (no error)"=w12) -> ("array out"=w8:string[])  [unwired: 8 in, 2 out]
  n10 = property on="run" class="Bool (strict)"(error in=w6, "Value"=TRUE ("run"), "Colors [4]"=cluster{u32, u32}[] [{6618880, 0}]) -> (error out=w19:errorcluster)  [unwired: 1 in, 1 out]
  n11 = Array To Cluster(array=w8) -> (cluster=w7:T11)
  n12 = while {
    shift-right: [w30] -> _
    shift-left: main_state_control."wait" -> [w52]
    shift-right: [w51] -> _
    shift-left: _ -> [w50]
    shift-right: [w48] -> _
    shift-left: _ -> [w47]
    shift-right: [w45] -> _
    shift-left: "stable data out 2" -> [w46]
    shift-right: [w27] -> _
    shift-left: w22 -> [w44]
    shift-right: [w43] -> _
    shift-left: w22 -> [w42]
    shift-right: [w28] -> _
    shift-left: "Measurement values" -> [w41]
    shift-right: [w40] -> _
    shift-left: "data out" -> [w39]
    shift-right: [w37] -> _
    shift-left: w7 -> [w38]
    tunnel: w19 -> [_]
    stop <- w53 stop-if-true
    n13 = shared-variable "My Computer\\SCA shared var - new.lvlib\\SCA Status"() -> (w24:T1)  [unwired: 1 in, 1 out]
    "SCA status" <- w24
    n14 = call "set gate shift.vi"("read write"=T12 "read") -> ()  [unwired: 10 in, 1 out]
    n15 = Equal?(x=SCA_broadcast_status."Sample change complete", y=w24) -> (x = y?=w26:bool)
    n16 = event shown="[0] Timeout" {
      selector: _ -> [_ _ _ _ _ _ _]
      dyn-events: _ -> [_ _ _ _ _ _ _]
      timeout: "time for each measurement" -> [_ _ _ _ _ _ _]
      tunnel: [FALSE _ FALSE FALSE FALSE FALSE FALSE] -> w53
      tunnel: w52 -> [w76 w520 _ _ _ _ _]
      tunnel: [w75 w520 main_state_control."insert cup" w595 main_state_control."wait" main_state_control."wait" main_state_control."wait"] -> w30
      tunnel: [w74 w530 w594 w606 w654 w670 w688] -> w51
      tunnel: w50 -> [w73 w530 w594 w606 w644 w660 w688]
      tunnel: [w68 w522 _ w603 w649 w661 w673] -> w49
      tunnel: [w71 w531 w593 w604 w651 w668 w672] -> w48
      tunnel: w47 -> [w71 w531 w593 w604 w651 w668 w680]
      tunnel: [w70 w532 w592 w602 w650 w667 w685] -> w45
      tunnel: w46 -> [w69 w532 w592 w602 w650 w667 w685]
      tunnel: [w67 u32 0 ("millisecond timer value") u32 0 ("millisecond timer value") u32 0 ("millisecond timer value") u32 0 ("millisecond timer value") u32 0 ("millisecond timer value") u32 0 ("millisecond timer value")] -> w27
      tunnel: w44 -> [w66 _ _ _ _ _ _]
      tunnel: [w65 _ _ _ _ _ _] -> w43
      tunnel: w42 -> [w64 _ _ _ _ _ _]
      tunnel: [w63 w525 w587 w597 w647 w665 w683] -> w28
      tunnel: w41 -> [w62 w526 w583 w598 w647 w665 w683]
      tunnel: [w61 w529 w590 w600 w646 w658 w682] -> w40
      tunnel: w39 -> [w60 w529 w590 w600 w646 w658 w682]
      tunnel: [w59 w523 w586 w599 w645 w664 w681] -> w37
      tunnel: w38 -> [w58 w524 w586 w599 w645 w664 w681]
      tunnel: w26 -> [w57 _ _ _ _ _ _]
      tunnel: "13 to 12 conversion .011 for 14C otherwise 1" -> [w56 _ _ _ _ _ _]
      tunnel: "time for each measurement" -> [w55 _ _ _ _ _ _]
      tunnel: "use SS ratio" -> [w54 _ _ _ _ _ _]
      event Timeout {
        n17 = event-data() -> ()  [unwired: 1 in, 2 out]
        n18 = case shown="\"check sample start\"" w76 {
          tunnel: [main_state_control."wait" main_state_control."wait" main_state_control."start rare" main_state_control."get rare" w137 main_state_control."get stable" main_state_control."get stable" main_state_control."check sample start" w258 w282 main_state_control."change sample" main_state_control."get transmission" w331 w436 main_state_control."check injector cup" main_state_control."record data"] -> w75
          tunnel: [w88 w89 w110 w111 w126 w179 w191 w205 w266 w274 w289 w315 w349 w363 w464 w484] -> w74
          tunnel: w73 -> [w88 w89 w110 w112 w127 w180 w192 w205 w266 w274 w289 w315 w349 w363 w464 w485]
          tunnel: w71 -> [_ _ _ _ _ _ _ _ _ _ _ _ _ _ w446 w517]
          tunnel: [w87 w100 w109 w125 w172 w190 w202 w208 w265 w273 w302 w314 w351 w362 w461 w480] -> w70
          tunnel: w69 -> [w87 w100 w109 w125 w172 w190 w202 w208 w265 w273 w302 w314 w351 w362 w469 w500]
          tunnel: [errorcluster {"status"=FALSE, "code"=0, "source"=""} ("error out") w91 errorcluster {"status"=FALSE, "code"=0, "source"=""} ("error out") w116 w148 w182 w201 w212 errorcluster {"status"=FALSE, "code"=0, "source"=""} ("error constant") w278 w294 w308 w348 w435 w448 w504] -> w68
          tunnel: [u32 0 ("millisecond timer value") u32 0 ("millisecond timer value") u32 0 ("millisecond timer value") w123 w150 w189 u32 100 ("millisecond timer value") w254 w264 w281 w301 w313 w316 w406 u32 1 ("millisecond timer value") w482] -> w67
          tunnel: w66 -> [_ _ _ w123 w150 w189 _ _ _ _ _ _ w316 w412 _ w482]
          tunnel: [w83 w97 w105 w122 w153 w187 w199 w209 w262 w271 w300 w311 w343 w433 w462 w483] -> w65
          tunnel: w64 -> [w83 w97 w105 w122 w153 w187 w199 w209 w262 w271 w300 w311 w343 w434 w462 w483]
          tunnel: [w84 w98 w106 w121 w164 w188 w200 w207 w263 w280 w288 w312 w317 w411 w455 w501] -> w63
          tunnel: w62 -> [w84 w98 w106 w121 w160 w188 w200 w207 w263 w280 w288 w312 w317 w405 w460 w481]
          tunnel: [w82 w96 w104 w120 w163 w186 w198 w206 w261 w279 w299 w310 w342 w404 w454 w499] -> w61
          tunnel: w60 -> [w82 w96 w104 w120 _ w186 w198 w206 w261 w279 w299 w310 w342 w404 w454 w499]
          tunnel: [w81 w95 w103 w115 w151 w185 w197 w241 w259 w272 w298 w309 w332 w361 w451 w498] -> w59
          tunnel: w58 -> [w81 w95 w103 w115 w154 w185 w197 _ w259 w272 w298 w309 w332 w361 w451 w498]
          tunnel: w57 -> [_ _ _ _ _ _ _ _ w260 _ _ _ _ _ _ _]
          tunnel: w56 -> [_ _ _ _ w129 _ _ _ _ _ _ _ _ _ _ w488]
          tunnel: w55 -> [_ _ _ _ _ _ _ _ _ _ _ _ _ _ _ _]
          tunnel: w54 -> [_ _ _ _ w135 _ _ _ _ _ _ _ _ _ _ w486]
          frame "wait", Default {
            w78 = u32 13816530
            # "wait"
            n19 = property on="run time(sec)" class="DigNum (strict)"("NumText.BGColor"=w78) -> (error out=w79:errorcluster)  [unwired: 2 in, 1 out]
            n20 = property on="sample warm up" class="DigNum (strict)"(error in=w79, "NumText.BGColor"=w78) -> ()  [unwired: 1 in, 2 out]
            n21 = property on="DAQ state control" class="Enum (strict)"("RingText.BGColor"=u32 16777238) -> ()  [unwired: 2 in, 2 out]
          }
          frame "set gate" {
            w92 = u32 13816530
            # "set gate"
            n22 = invoke class="VI" method="Abort VI"(reference=w89) -> (error out=w91:errorcluster)  [unwired: 2 in, 2 out]
            n23 = property on="DAQ state control" class="Enum (strict)"("RingText.BGColor"=u32 16777238) -> ()  [unwired: 2 in, 2 out]
            n24 = property on="run time(sec)" class="DigNum (strict)"("NumText.BGColor"=w92) -> (error out=w93:errorcluster)  [unwired: 2 in, 1 out]
            n25 = property on="sample warm up" class="DigNum (strict)"(error in=w93, "NumText.BGColor"=w92) -> ()  [unwired: 1 in, 2 out]
          }
          frame "check injector cup" {
            # "check injector cup"
            n26 = property on="DAQ state control" class="Enum (strict)"("RingText.BGColor"=u32 16711680) -> ()  [unwired: 2 in, 2 out]
          }
          frame "start rare" {
            w124 = FALSE ("Auto Dispose Reference")
            # "start rare"
            n27 = property on="DAQ state control" class="Enum (strict)"("RingText.BGColor"=u32 4194090) -> ()  [unwired: 2 in, 2 out]
            n28 = invoke class="VI" method="Run VI"(reference=w112, "Wait until done"=w124, "Auto Dispose Ref"=w124) -> (reference out=w111:refnum<vi>, error out=w117:errorcluster)  [unwired: 2 in, 3 out]
            n29 = property on="run time(sec)" class="DigNum (strict)"("NumText.BGColor"=u32 6618880) -> ()  [unwired: 2 in, 2 out]
            n30 = call "Time Delay"("error in (no error)"=w117) -> ("error out"=w116:errorcluster)  [unwired: 10 in]
            n31 = local write "sample change failure"(u32 16777238 ("sample change failure")) -> ()
          }
          frame "get rare" {
            # "get rare"
            n32 = Number To Decimal String(number=w150) -> (decimal integer string=w152:string)  [unwired: 1 in]
            n33 = Bundle By Name(cluster=w154, "array out[4]"=w152) -> (w151:T11)
            n34 = invoke class="VI" method="Ctrl Val.Set"(reference=w127, "Control Name"="1d state control", "Value"="get data" ("Control Name")) -> (reference out=w171:refnum<vi>, error out=w170:errorcluster)  [unwired: 2 in, 3 out]
            n35 = Unbundle By Name(w160) -> ("SS Injector"=w128:dbl, "2nd Current 1"=w159:dbl, "Current 1"=w158:dbl)
            n36 = invoke class="VI" method="Ctrl Val.Get"(reference=w171, error in=w170, "Control Name"="data out") -> (reference out=w126:refnum<vi>, error out=w168:errorcluster, "Get Control Value Variant"=w175:variant)  [unwired: 1 in, 1 out]
            n37 = Variant To Data(error in=w168, type=T7 {"Total counts"=2112, "cps"=59.881992625371424, "live time"=1.0009469696969697, "pulser"=2114.0, "rare counts"=2112.0, "other counts"=4294965182.0, "total run time(sec)"=35.236, "adjusted run time(sec)"=35.269367424242425, "17O average"=1.0, "17O current"=1.0} ("data out"), Variant=w175) -> (data=w163:T7, error out=w149:errorcluster)
            n38 = Unbundle By Name(w163) -> ("adjusted run time(sec)"=w155:dbl, "total run time(sec)"=w131:dbl, "cps"=w167:dbl, "live time"=w162:dbl, "rare counts"=w144:dbl, "17O current"=w142:dbl)
            "run time(sec)" <- w131
            n39 = shared-variable "My Computer\\CONnie shared var.lvlib\\rare count rate"(error in=w149) -> (→"rare count rate":dbl, error out=w148:errorcluster)
            n40 = call "Pixie4ReadRunStatistics.vi"() -> ("run data output"=w146:T6)  [unwired: 8 in, 3 out]
            "run data output" <- w146
            n41 = call "stable error and currents.vi"("Charge State"="Charge State", "ss ratio 2"=w135, "ss ratio"=w128, "Stable Current 1"=w159, "Stable Current 2"=w158, "Live Time"=w155) -> ("Stable Counts"=w157:dbl)  [unwired: 8 in, 1 out]
            n42 = Divide(x=w144, y=w142) -> (x/y=w143:dbl)
            n43 = call "cycle ratio.vi"("Stable Counts"=w157, "rare Counts"=w144) -> ("Cycle ratio"=w130:dbl)
            n44 = Multiply(x=w129, y=w130) -> (x*y=w156:dbl)
            n45 = Unbundle By Name(w146) -> ("number of events"=w145:dbl, "event rate"=w141:dbl, "input count rate 0"=→"input count rate 0":dbl)
            n46 = Greater Or Equal?(x=w131, y="run time") -> (x >= y?=w173:bool)
            n47 = Greater Or Equal?(x=w141, y="abort count rate (cps)") -> (x >= y?=w139:bool)
            n48 = Select(t=main_state_control."stop rare", s=w173, f=main_state_control."get rare") -> (s? t:f=w138:T2)
            n49 = Multiply(x=w167, y=60.0) -> (x*y=w165:dbl)
            n50 = Bundle By Name(cluster=w160, "rare/stable"=w156, "run time"=w131, "Counts"=w144, "Live Time"=w162, "Counts per minute"=w165, "Interference rate(cps"=w141, "total interference counts"=w145, "10Be vs O17"=w143, "O17 cycle Error"=w142) -> (w164:T8)
            n51 = Select(t=main_state_control."abort run", s=w139, f=w138) -> (s? t:f=w137:T2)
          }
          frame "stop rare" {
            # "stop rare"
            n52 = property on="DAQ state control" class="Enum (strict)"("RingText.BGColor"=u32 3381759) -> ()  [unwired: 2 in, 2 out]
            n53 = property on="run time(sec)" class="DigNum (strict)"("NumText.BGColor"=u32 13816530) -> ()  [unwired: 2 in, 2 out]
            n54 = invoke class="VI" method="Abort VI"(reference=w180) -> (reference out=w179:refnum<vi>, error out=w182:errorcluster)  [unwired: 2 in, 1 out]
          }
          frame "abort run" {
            # "abort run"
            n55 = property on="DAQ state control" class="Enum (strict)"("RingText.BGColor"=u32 3381759) -> ()  [unwired: 2 in, 2 out]
            n56 = property on="run time(sec)" class="DigNum (strict)"("NumText.BGColor"=u32 13816530) -> ()  [unwired: 2 in, 2 out]
            n57 = invoke class="VI" method="Abort VI"(reference=w192) -> (reference out=w191:refnum<vi>, error out=w201:errorcluster)  [unwired: 2 in, 1 out]
          }
          frame "change sample" {
            # "change sample"
            n58 = property on="DAQ state control" class="Enum (strict)"("RingText.BGColor"=u32 16746562) -> ()  [unwired: 2 in, 2 out]
            n59 = call "shift wheel.vi"("read write"="read") -> ("cycle results name out"=w243:path, "Group run list"=w251:string[][], "seq results name out"=w242:path)  [unwired: 8 in]
            n60 = call "get current index.vi"("Group run list in"=w251) -> ("current index"=w248:i32)  [unwired: 8 in, 2 out]
            n61 = Replace Array Subset(array=w251, new element="Finished", index (row)=w248, index (col)=7 ("disabled index (col)")) -> (w215:string[][])
            n62 = Index Array(array=w215, index (row)=w248) -> (element=w247:string[])  [unwired: 1 in]
            n63 = call "shift wheel.vi"("seq results name in"=w242, "cycle results name in"=w243, "Group run list write"=w215, "read write"="Write") -> ("Group run list"=w240:string[][])  [unwired: 5 in, 2 out]
            n64 = Index Array(array=w247, index=0) -> (element=w229:string)
            n65 = Decimal String To Number(string=w229) -> (number=w244:i32)  [unwired: 2 in, 1 out]
            "sample number" <- w244
            n66 = call "sort sample information.vi"("Group run list write"=w240) -> ("array out"=w245:string[], "error out"=w203:errorcluster)  [unwired: 8 in, 1 out]
            n67 = shared-variable "My Computer\\SCA shared var - new.lvlib\\Requested Sample"(w244, error in=w203) -> (error out=w214:errorcluster)
            n68 = local read "wheelnumber"() -> (w232:string)
            n69 = local read "run number"() -> (w234:string)
            n70 = call <vilib>:"Space Constant.vi"() -> ("String"=w231:string)
            n71 = call "Time Delay2"("error in (no error)"=w214) -> ("error out"=w213:errorcluster)  [unwired: 10 in]
            n72 = Concatenate Strings("select distinct position from cycleresults where runnumber=" ("SQL query"), w234, w231, "and wheelnumber=" ("string"), w232, w231, "and position=" ("string"), w229, ";" ("string")) -> (w227:string)
            n73 = call-poly <vilib>:"DB Tools Open Connection.vi"("connection information"="amsrecord") -> ("error out"=w236:errorcluster, "connection reference"=w237:T15)  [unwired: 7 in]
            n74 = call-poly <vilib>:"DB Tools Execute Query.vi"("error in (no error)"=w236, "SQL query"=w227, "connection reference"=w237) -> ("error out"=w226:errorcluster, "recordset reference"=w225:T16)  [unwired: 5 in]
            n75 = call-poly <vilib>:"DB Tools Fetch Recordset Data.vi"("error in (no error)"=w226, "recordset reference"=w225) -> ("error out"=w224:errorcluster, "recordset data"=w211:variant[][], "recordset reference out"=w223:T16)  [unwired: 3 in]
            "recordset data" <- w211
            n76 = call-poly <vilib>:"DB Tools Free Object.vi"("error in (no error)"=w224, "recordset reference"=w223) -> ("error out"=w217:errorcluster, "connection reference"=w218:T15)  [unwired: 8 in]
            n77 = Array Size(array=w211) -> (size(s)=w222:i32[])
            n78 = shared-variable "My Computer\\SCA shared var - new.lvlib\\SM Command"(SCA_commands."Start sample change" ("SM Command"), error in=w213) -> (error out=w212:errorcluster)
            n79 = call <vilib>:"DB Tools Close Connection.vi"("error in (no error)"=w217, "connection reference"=w218) -> ("error out"=→"Sample DB fetch error":errorcluster)  [unwired: 5 in]
            n80 = Index Array(array=w222, index=0) -> (element=w220:i32)
            n81 = Equal To 0?(x=w220) -> (x = 0?=→"first time run":bool)
            n82 = Tick Count (ms)() -> (millisecond timer value=w254:u32)
            n83 = Array To Cluster(array=w245) -> (cluster=w241:T11)
          }
          frame "wait for sample change" {
            # "wait for sample change"
            n84 = Select(t=main_state_control."sample warm up", s=w260, f=main_state_control."wait for sample change") -> (s? t:f=w258:T2)
            n85 = Tick Count (ms)() -> (millisecond timer value=w264:u32)
          }
          frame "check sample start" {
            # "check sample start"
            n86 = shared-variable "My Computer\\SCA shared var - new.lvlib\\SCA Status"() -> (w269:T1, error out=w267:errorcluster)  [unwired: 1 in]
            "Sample Change Start SV error" <- w267
            n87 = Equal?(x=SCA_broadcast_status."Changing samples", y=w269) -> (x = y?=w268:bool)
            n88 = call <vilib>:"Clear Errors.vi"("error in (no error)"=w267) -> ("error out"=w277:errorcluster)  [unwired: 5 in, 1 out]
            n89 = call "Time Delay8"("error in (no error)"=w277) -> ("error out"=w278:errorcluster)  [unwired: 10 in]
            n90 = case shown="False" w268 {
              tunnel: [w284 errorcluster {"status"=FALSE, "code"=0, "source"=""} ("error IO")] -> _
              frame False {
                n91 = local read "sample number"() -> (w285:u16)
                n92 = shared-variable "My Computer\\SCA shared var - new.lvlib\\Requested Sample"(w285) -> (error out=w286:errorcluster)  [unwired: 1 in]
                n93 = shared-variable "My Computer\\SCA shared var - new.lvlib\\SM Command"(SCA_commands."Start sample change" ("SM Command"), error in=w286) -> (error out=w284:errorcluster)
              }
              frame True {
              }
            }
            n94 = Select(t=main_state_control."wait for sample change", s=w268, f=main_state_control."check sample start") -> (s? t:f=w282:T2)
            n95 = Tick Count (ms)() -> (millisecond timer value=w281:u32)
          }
          frame "insert cup" {
            # "insert cup"
            n96 = Tick Count (ms)() -> (millisecond timer value=w301:u32)
            n97 = shared-variable "My Computer\\InjA-Image shared var.lvlib\\injector cup"(FALSE ("turn cathode on")) -> (error out=w292:errorcluster)  [unwired: 1 in]
            n98 = shared-variable "My Computer\\LowEnd shared var.lvlib\\LE waist cup"(FALSE ("LE waist cup"), error in=w292) -> (error out=w291:errorcluster)
            n99 = shared-variable "My Computer\\DAQuiri shared var.lvlib\\sample change complete"(FALSE ("s"), error in=w291) -> (error out=w295:errorcluster)
            n100 = call "Time Delay5"("error in (no error)"=w295) -> ("error out"=w294:errorcluster)  [unwired: 10 in]
          }
          frame "remove cup" {
            # "remove cup"
            n101 = shared-variable "My Computer\\InjA-Image shared var.lvlib\\injector cup"(TRUE ("turn cathode on")) -> (error out=w306:errorcluster)  [unwired: 1 in]
            n102 = shared-variable "My Computer\\LowEnd shared var.lvlib\\LE waist cup"(TRUE ("LE waist cup"), error in=w306) -> (error out=w305:errorcluster)
            n103 = call "Time Delay6"("error in (no error)"=w305) -> ("error out"=w308:errorcluster)  [unwired: 10 in]
            n104 = Tick Count (ms)() -> (millisecond timer value=w313:u32)
          }
          frame "sample warm up" {
            w350 = FALSE ("Auto Dispose Reference")
            # "sample warm up"
            n105 = Unbundle By Name(w332) -> ("array out[5]"=w324:string)
            n106 = shared-variable "My Computer\\SCA shared var - new.lvlib\\Requested Sample"() -> (w328:u8)  [unwired: 1 in, 1 out]
            "change sample" <- w328
            n107 = Tick Count (ms)() -> (millisecond timer value=w347:u32)
            n108 = Subtract(x=w347, y=w316) -> (x-y=w346:u32)
            n109 = Decimal String To Number(string=w324, default (0L)=u8 0 ("default (0 I32)")) -> (offset past number=w327:i32)  [unwired: 1 in, 1 out]
            n110 = Divide(x=w346, y=u32 1000) -> (x/y=w345:dbl)
            "sample warm up" <- w345
            n111 = Equal?(x=w324, y="1") -> (x = y?=w322:bool)
            n112 = Equal?(x=w328, y=w327) -> (x = y?=w325:bool)
            n113 = invoke class="VI" method="Run VI"(reference=w349, "Wait until done"=w350, "Auto Dispose Ref"=w350) -> (error out=w348:errorcluster)  [unwired: 2 in, 4 out]
            n114 = Not(x=w325) -> (.not. x?=w329:bool)
            n115 = local read "first time run"() -> (w336:bool)
            n116 = property on="run time(sec)" class="DigNum (strict)"("NumText.BGColor"=u32 13816530) -> (error out=w340:errorcluster)  [unwired: 2 in, 1 out]
            n117 = Select(t=u32 32639, s=w336, f=u32 16746562) -> (s? t:f=w333:u32)
            n118 = Select(t="1st sample warm up time", s=w336, f="2nd sample warm up time 2") -> (s? t:f=w338:dbl)
            n119 = property on="sample warm up" class="DigNum (strict)"(error in=w340, "NumText.BGColor"=w333) -> ()  [unwired: 1 in, 2 out]
            n120 = Greater Or Equal?(x=w338, y=w345) -> (x >= y?=w321:bool)
            n121 = Or(x=w322, y=w321) -> (x .or. y?=w320:bool)
            n122 = Select(t=main_state_control."sample warm up", s=w321, f=main_state_control."remove cup") -> (s? t:f=w330:T2)
            n123 = case shown="False" w320 {
              tunnel: w329 -> [w354 _]
              tunnel: [w355 w359] -> w331
              tunnel: w330 -> [w353 w359]
              frame False {
                n124 = Select(t=u32 16777238 ("sample change failure"), s=w354, f=u32 14418097 ("sample change failure")) -> (s? t:f=w356:u32)
                n125 = local write "sample change failure"(w356) -> ()
                n126 = Select(t=w353, s=w354, f=main_state_control."wait") -> (s? t:f=w355:T2)
              }
              frame True {
              }
            }
          }
          frame "record data" {
            w372 = "\r"
            # "record data"
            n127 = Increment(x=w434) -> (x+1=w433:u32)
            n128 = Unbundle By Name(w405) -> ("Cycle number"=w410:dbl)
            n129 = Unbundle By Name(w404) -> ("pulser"=w432:dbl, "Total counts"=w430:u32, "17O current"=w431:dbl, "other counts"=w427:dbl, "total run time(sec)"=w429:dbl, "adjusted run time(sec)"=w428:dbl, "17O average"=w425:dbl)  [unwired: 1 out]
            n130 = Current VI's Path() -> (path=w403:path)
            n131 = Open VI Reference(vi path=w403) -> (vi reference=w402:refnum<vi>, error out=w400:errorcluster)  [unwired: 5 in]
            n132 = Cluster To Array(cluster=w405) -> (array=w421:dbl[])
            n133 = Increment(x=w410) -> (x+1=w409:dbl)
            n134 = invoke class="VI" method="Ctrl Val.Get All"(reference=w402, error in=w400, "Controls"=TRUE) -> (reference out=w401:refnum<vi>, "Get All Control Values Variant"=w389:cluster{"Name":string, "Variant Data":variant}[])  [unwired: 1 in, 2 out]
            n135 = Bundle By Name(cluster=w405, "Cycle number"=w409) -> (w411:T8)
            n136 = local read "input count rate 0"() -> (w368:dbl)
            n137 = Close Reference(reference=w401) -> ()  [unwired: 1 in, 1 out]
            n138 = Divide(x=w427, y=w428) -> (x/y=w426:dbl)
            n139 = for {
              tunnel: w389 -> [w443] mode=indexing
              tunnel: [w441] -> w388 mode=indexing
              tunnel: [w437] -> _ mode=indexing
              n140 = Unbundle By Name(w443) -> ("Name"=w442:string, "Variant Data"=w439:variant)
              n141 = Variant To Flattened String(Variant=w439) -> (data string=w438:string, 1:w437:i16[])
              n142 = Build Array(w442, "\t", w438) -> (w441:string[])
            }
            n143 = Build Array(w432, w431, w430, w427, w429, w428, w368, w426, w426, w426, w425) -> (w420:dbl[])
            n144 = Build Array (concatenate)(w421, w420) -> (w423:dbl[])
            n145 = Current VI's Path() -> (path=w398:path)
            n146 = Strip Path(path=w398) -> (stripped path=w397:path)  [unwired: 1 out]
            n147 = Build Path(base path=w397, name or relative path="cycle.txt") -> (appended path=w395:path)
            n148 = Array To Spreadsheet String(array=w423, 3:"" ("format string")) -> (spreadsheet string=w422:string)  [unwired: 1 in]
            n149 = property on="DAQ state control" class="Enum (strict)"("RingText.BGColor"=u32 16776704) -> (error out=w360:errorcluster)  [unwired: 2 in, 1 out]
            n150 = Array To Spreadsheet String(delimiter (Tab)=",", array=w388, 3:"" ("format string")) -> (spreadsheet string=w385:string)
            n151 = Open/Create/Replace File(file path (use dialog)=w395, operation (0:open)=T14."replace or create") -> (refnum out=w393:refnum<file>, error out=w392:errorcluster)  [unwired: 4 in, 1 out]
            n152 = Write to Text File(file (use dialog)=w393, text=w385, error in=w392) -> (refnum out=w391:refnum<file>, error out=w390:errorcluster)  [unwired: 1 in, 1 out]
            n153 = call "sort sample information.vi"() -> ("spreadsheet string"=w419:string)  [unwired: 9 in, 2 out]
            n154 = Close File(refnum=w391, error in=w390) -> ()  [unwired: 2 out]
            n155 = call "shift wheel.vi"("read write"="read") -> ("cycle results name out"=w375:path, "seq results name out"=w374:path)  [unwired: 8 in, 1 out]
            n156 = call "cycle writer.vi"("wheel name"=w375, "error in"=w360, "Cycle data"=w422, "Wheel data"=w419) -> ("error out"=w435:errorcluster, "readouts string"=w414:string)  [unwired: 6 in]
            n157 = Current VI's Path() -> (path=w376:path)
            n158 = Path To String(path=w375) -> (string=w373:string)
            n159 = Path To String(path=w374) -> (string=w370:string)
            n160 = Strip Path(path=w376) -> (stripped path=w377:path)  [unwired: 1 out]
            n161 = Build Path(base path=w377, name or relative path="wheel.txt") -> (appended path=w379:path)
            n162 = shared-variable "My Computer\\DAQuiri shared var.lvlib\\wheel folder"() -> (w371:string)  [unwired: 1 in, 1 out]
            n163 = call "database input.vi"("Wheel Name"="Wheel Name", "run number"="run number", "wheelnumber"="wheelnumber", "readouts string"=w414, "runletter"="runletter") -> ("error out"=→"DB input error":errorcluster)  [unwired: 5 in, 1 out]
            n164 = Open/Create/Replace File(file path (use dialog)=w379, operation (0:open)=T14."replace or create") -> (refnum out=w381:refnum<file>, error out=w382:errorcluster)  [unwired: 4 in, 1 out]
            n165 = Concatenate Strings(w373, w372, w370, w372, w371) -> (w369:string)
            n166 = Write to Text File(file (use dialog)=w381, text=w369, error in=w382) -> (refnum out=w383:refnum<file>, error out=w384:errorcluster)  [unwired: 1 in, 1 out]
            n167 = Increment(x=w412) -> (x+1=w406:u32)
            n168 = Close File(refnum=w383, error in=w384) -> ()  [unwired: 2 out]
            n169 = Greater Or Equal?(x=w406, y="number of cycles") -> (x >= y?=w367:bool)
            n170 = Select(t=main_state_control."insert cup", s=w367, f=main_state_control."start rare") -> (s? t:f=w436:T2)
          }
          frame "get transmission" {
            # "get transmission"
            n171 = invoke class="VI" method="Abort VI"(reference=w464) -> (error out=w453:errorcluster)  [unwired: 2 in, 2 out]
            n172 = call <vilib>:"Clear Errors.vi"("error in (no error)"=w453) -> ("error out"=w452:errorcluster)  [unwired: 5 in, 1 out]
            n173 = property on="DAQ state control" class="Enum (strict)"("RingText.BGColor"=u32 3381759) -> ()  [unwired: 2 in, 2 out]
            n174 = property on="sample warm up" class="DigNum (strict)"("NumText.BGColor"=u32 13816530) -> ()  [unwired: 2 in, 2 out]
            n175 = invoke class="VI" method="Ctrl Val.Set"(reference=w446, error in=w452, "Control Name"="stable data in", "Value"=w469) -> (reference out=w472:refnum<vi>, error out=w465:errorcluster)  [unwired: 1 in, 3 out]
            n176 = invoke class="VI" method="Ctrl Val.Set"(reference=w472, error in=w465, "Control Name"="measure transmission?", "Value"=TRUE ("Wait Until Done")) -> (reference out=w471:refnum<vi>, error out=w467:errorcluster)  [unwired: 1 in, 3 out]
            n177 = invoke class="VI" method="Run VI"(reference=w471, error in=w467, "Wait until done"=TRUE ("Wait Until Done"), "Auto Dispose Ref"=FALSE ("Auto Dispose Reference")) -> (reference out=w476:refnum<vi>, error out=w468:errorcluster)  [unwired: 1 in, 3 out]
            n178 = invoke class="VI" method="Ctrl Val.Get"(reference=w476, error in=w468, "Control Name"="stable data out") -> (error out=w466:errorcluster, "Get Control Value Variant"=w474:variant)  [unwired: 1 in, 2 out]
            n179 = Variant To Data(error in=w466, type=w469, Variant=w474) -> (data=w461:T10, error out=w449:errorcluster)
            n180 = call "Time Delay4"("error in (no error)"=w449) -> ("error out"=w448:errorcluster)  [unwired: 10 in]
            n181 = Unbundle By Name(w461) -> ("transmission"=w458:dbl, "ss inj ratio"=w456:dbl, "ss offset ratio"=w457:dbl, "offset current"=w459:dbl)
            n182 = Bundle By Name(cluster=w460, "SS Injector"=w456, "SS High End"=w457, "Transmission"=w458, "2nd Current 1"=w459, "Current 1"=w459) -> (w455:T8)
          }
          frame "get stable" {
            # "get stable"
            # "Sets some fo the controls in the stable data VI, runs it, gets the data out of it."
            n183 = local write "data out"(w499) -> ()
            n184 = invoke class="VI" method="Abort VI"(reference=w485) -> (reference out=w484:refnum<vi>, error out=w503:errorcluster)  [unwired: 2 in, 1 out]
            n185 = local write "Measurement values"(w481) -> ()
            n186 = local write "stable data out 2"(w500) -> ()
            n187 = call <vilib>:"Clear Errors.vi"("error in (no error)"=w503) -> ("error out"=w502:errorcluster)  [unwired: 5 in, 1 out]
            n188 = invoke class="VI" method="Ctrl Val.Set"(reference=w517, error in=w502, "Control Name"="stable data in", "Value"=w500) -> (reference out=w511:refnum<vi>, error out=w506:errorcluster)  [unwired: 1 in, 3 out]
            n189 = invoke class="VI" method="Ctrl Val.Set"(reference=w511, error in=w506, "Control Name"="measure transmission?", "Value"=FALSE ("Wait Until Done")) -> (reference out=w510:refnum<vi>, error out=w508:errorcluster)  [unwired: 1 in, 3 out]
            n190 = invoke class="VI" method="Run VI"(reference=w510, error in=w508, "Wait until done"=TRUE ("Wait Until Done"), "Auto Dispose Ref"=FALSE ("Auto Dispose Reference")) -> (reference out=w516:refnum<vi>, error out=w507:errorcluster)  [unwired: 1 in, 3 out]
            n191 = invoke class="VI" method="Ctrl Val.Get"(reference=w516, error in=w507, "Control Name"="stable data out") -> (error out=w505:errorcluster, "Get Control Value Variant"=w514:variant)  [unwired: 1 in, 2 out]
            n192 = Unbundle By Name(w481) -> ("Current 1"=w493:dbl, "Counts"=w496:dbl, "SS Injector"=w492:dbl, "run time"=w491:dbl)
            n193 = Variant To Data(error in=w505, type=w500, Variant=w514) -> (data=w480:T10, error out=w504:errorcluster)
            n194 = Unbundle By Name(w480) -> ("offset current"=w494:dbl, "ss offset ratio"=w497:dbl)
            n195 = local read "Charge State"() -> (w495:dbl)
            n196 = call "stable error and currents.vi"("Charge State"=w495, "ss ratio 2"=w486, "ss ratio"=w492, "Stable Current 1"=w494, "Stable Current 2"=w493, "Live Time"=w491) -> ("Stable Counts"=w490:dbl)  [unwired: 8 in, 1 out]
            n197 = call "cycle ratio.vi"("Stable Counts"=w490, "rare Counts"=w496) -> ("Cycle ratio"=w489:dbl)
            n198 = Multiply(x=w489, y=w488) -> (x*y=w487:dbl)
            n199 = Bundle By Name(cluster=w481, "Current 1"=w494, "2nd Current 1"=w493, "SS High End"=w497, "rare/stable"=w487) -> (w501:T8)
          }
        }
      }
      event Menu Selection (User) {
        n200 = event-data() -> ("ItemTag"=w521:string)  [unwired: 1 in, 5 out]
        n201 = Unbundle By Name(w526) -> ("Cycle number"=w528:dbl)
        n202 = case shown="\"save pixie parameters\"" w521 {
          tunnel: [errorcluster {"status"=FALSE, "code"=0, "source"=""} ("error out") w539 errorcluster {"status"=FALSE, "code"=0, "source"=""} ("error out") errorcluster {"status"=FALSE, "code"=0, "source"=""} ("error out") errorcluster {"status"=FALSE, "code"=0, "source"=""} ("error out") w559] -> w522
          tunnel: w528 -> [w534 w537 w545 w549 w556 w565]
          tunnel: [w534 w537 w545 w549 w556 w564] -> w527
          tunnel: w524 -> [w535 w541 w543 w547 w554 _]
          tunnel: [w535 w541 w543 w547 w554 w562] -> w523
          frame "False", Default {
          }
          frame "reboot" {
            # "Reboots Pixie4: asks for DSP file to use, along with crate and slot location of Pixie4"
            n203 = call "preload default boot.vi"() -> ("PreLoad error"=w540:errorcluster, "BootFile error"=w538:errorcluster)  [unwired: 10 in]
            n204 = Merge Errors(w538, w540) -> (w539:errorcluster)
          }
          frame "set pixie parameters" {
            n205 = vi-ref "Pixie4SetUserPar.vi"() -> (w542:refnum<vi>)
            n206 = invoke class="VI" method="FP.Open"(reference=w542) -> ()  [unwired: 4 in, 5 out]
          }
          frame "High speed stable" {
            n207 = vi-ref "stable test.vi"() -> (w546:refnum<vi>)
            n208 = invoke class="VI" method="FP.Open"(reference=w546) -> ()  [unwired: 4 in, 5 out]
          }
          frame "save pixie parameters" {
            n209 = vi-ref "Pixie4SaveDSPParToFile.vi"() -> (w553:refnum<vi>)
            n210 = invoke class="VI" method="FP.Open"(reference=w553) -> (reference out=w552:refnum<vi>)  [unwired: 4 in, 4 out]
            n211 = invoke class="VI" method="Run VI"(reference=w552, "Wait until done"=FALSE ("Wait Until Done"), "Auto Dispose Ref"=TRUE ("Auto Dispose Reference")) -> ()  [unwired: 2 in, 5 out]
          }
          frame "change wheel" {
            n212 = property on="wheelnumber" class="Str"() -> ("Value"=w569:string)  [unwired: 2 in, 2 out]
            n213 = property on="run number" class="Str"() -> ("Value"=w558:string)  [unwired: 2 in, 2 out]
            n214 = property on="runletter" class="Str"() -> ("Value"=w572:string)  [unwired: 2 in, 2 out]
            n215 = Decimal String To Number(string=w569) -> (number=w568:i32)  [unwired: 2 in, 1 out]
            n216 = call "popupwheel.vi"("run number"=w558, "runletter"=w572, "Wheel Number"=w568) -> ("run number out"=w557:string, "runletter out"=w567:string, "Wheel Number  out"=w571:string, "New Wheel Location 2"=w573:path, "Wheel Name"=w570:string)  [unwired: 4 in]
            n217 = property on="run number" class="Str"("Value"=w557) -> ()  [unwired: 2 in, 2 out]
            n218 = property on="wheelnumber" class="Str"("Value"=w571) -> ()  [unwired: 2 in, 2 out]
            n219 = call "load wheel.vi"("file path"=w573) -> ("error out"=w561:errorcluster, "Wheel run order array"=→"Wheel run order array":string[][])  [unwired: 7 in, 2 out]
            n220 = property on="Wheel Name" class="Str"("Value"=w570) -> ()  [unwired: 2 in, 2 out]
            n221 = Equal?(x=w558, y=w557) -> (x = y?=w566:bool)
            n222 = property on="runletter" class="Str"(error in=w561, "Value"=w567) -> (error out=w560:errorcluster)  [unwired: 1 in, 1 out]
            n223 = case shown="True" w566 {
              tunnel: w565 -> [w575 w582]
              tunnel: [w577 w582] -> w564
              frame False {
                n224 = Two Button Dialog(message="The run letter has changed,\nwould you like to reset the cycle number?", 1:"no" ("F button name (\"Cancel\")"), 2:"yes" ("T button name (\"OK\")")) -> (T button?=w578:bool)
                n225 = Select(t=0.0 ("f"), s=w578, f=w575) -> (s? t:f=w577:dbl)
              }
              frame True {
              }
            }
            n226 = call "sort sample information.vi"("error in (no error)"=w560) -> ("array out"=w563:string[], "error out"=w559:errorcluster)  [unwired: 8 in, 1 out]
            n227 = Array To Cluster(array=w563) -> (cluster=w562:T11)
          }
        }
        n228 = Bundle By Name(cluster=w526, "Cycle number"=w527) -> (w525:T8)
      }
      event "skip sample": Value Change {
        n229 = event-data() -> ()  [unwired: 1 in, 1 out]
        n230 = Unbundle By Name(w583) -> ("Cycle number"=w589:dbl)
        n231 = Increment(x=w589) -> (x+1=w588:dbl)
        n232 = Bundle By Name(cluster=w583, "Cycle number"=w588) -> (w587:T8)
      }
      event "run": Value Change {
        n233 = event-data() -> ("NewVal"=w596:bool)  [unwired: 1 in, 4 out]
        n234 = case shown="False" w596 {
          tunnel: w606 -> [_ w634]
          tunnel: [w610 w631] -> w603
          tunnel: w598 -> [w607 w628]
          tunnel: [w611 w628] -> w597
          tunnel: [main_state_control."remove cup" main_state_control."wait"] -> w595
          frame False {
            # "Starting Run"
            n235 = property on="run" class="Bool (strict)"("Colors [4]"=cluster{u32, u32}[] [{16711680, 0}]) -> ()  [unwired: 2 in, 2 out]
            n236 = call "shift wheel.vi"("read write"="read") -> ("cycle results name out"=w614:path)  [unwired: 8 in, 2 out]
            n237 = call <vilib>:"Check if File or Folder Exists.vi"("path"=w614) -> ("error out"=w610:errorcluster, "file or folder exists?"=w613:bool, "dup path"=w612:path)  [unwired: 8 in]
            n238 = case shown="True" w613 {
              tunnel: w612 -> [_ w627]
              tunnel: w607 -> [w616 w623]
              tunnel: [w616 w622] -> w611
              frame False {
              }
              frame True {
                n239 = call-poly <vilib>:"Read Delimited Spreadsheet.vi"("file path (dialog if empty)"=w627) -> ("all rows"=w626:dbl[][])  [unwired: 9 in, 5 out]
                n240 = Index Array(array=w626, index (col)=8 ("disabled index (col)")) -> (element=w619:dbl[])  [unwired: 1 in]
                n241 = Reverse 1D Array(array=w619) -> (reversed array=w621:dbl[])
                n242 = Index Array(array=w621, index=0) -> (element=w618:dbl)
                n243 = Add(x=w618, y=5.0) -> (x+y=w617:dbl)
                n244 = Bundle By Name(cluster=w623, "Cycle number"=w617) -> (w622:T8)
              }
            }
          }
          frame True {
            w637 = FALSE ("Auto Dispose Reference")
            # "Pausing Run"
            n245 = property on="run" class="Bool (strict)"("Colors [4]"=cluster{u32, u32}[] [{6618880, 0}]) -> ()  [unwired: 2 in, 2 out]
            n246 = invoke class="VI" method="Ctrl Val.Set"(reference=w634, "Control Name"="1d state control", "Value"="stop" ("Control Name")) -> (reference out=w636:refnum<vi>, error out=w632:errorcluster)  [unwired: 2 in, 3 out]
            n247 = invoke class="VI" method="Run VI"(reference=w636, error in=w632, "Wait until done"=w637, "Auto Dispose Ref"=w637) -> (error out=w631:errorcluster)  [unwired: 1 in, 4 out]
          }
        }
      }
      event Value Change {
        w641 = FALSE ("Wait Until Done")
        n248 = event-data() -> ()  [unwired: 1 in, 6 out]
        n249 = case shown="\"2d\"" "Rare Event Data" {
          tunnel: [w655 w656 w657] -> w640
          frame "1d" {
            n250 = vi-ref "1d.vi"() -> (w655:refnum<vi>)
          }
          frame "2d 10Be" {
            n251 = vi-ref "2d 10Be.vi"() -> (w656:refnum<vi>)
          }
          frame "2d" {
            n252 = vi-ref "2d.vi"() -> (w657:refnum<vi>)
          }
        }
        n253 = invoke class="VI" method="Abort VI"(reference=w644) -> (error out=w643:errorcluster)  [unwired: 2 in, 2 out]
        n254 = call <vilib>:"Clear Errors.vi"("error in (no error)"=w643) -> ("error out"=w642:errorcluster)  [unwired: 5 in, 1 out]
        n255 = invoke class="VI" method="Run VI"(reference=w640, error in=w642, "Wait until done"=w641, "Auto Dispose Ref"=w641) -> (reference out=w654:refnum<vi>, error out=w652:errorcluster)  [unwired: 1 in, 3 out]
        "Rare Event Window error" <- w652
        n256 = invoke on="rare event display" class="SubPanel" method="Insert VI"(error in=w652, "VI Ref"=w654) -> (error out=w649:errorcluster)  [unwired: 2 in, 3 out]
      }
      event "reset": Value Change {
        n257 = event-data() -> ()  [unwired: 1 in, 1 out]
        n258 = invoke class="VI" method="Abort VI"(reference=w660) -> (error out=w663:errorcluster)  [unwired: 2 in, 2 out]
        n259 = call <vilib>:"Clear Errors.vi"("error in (no error)"=w663) -> ("error out"=w662:errorcluster)  [unwired: 5 in, 1 out]
        n260 = invoke class="VI" method="Run VI"(reference=w660, error in=w662, "Wait until done"=FALSE ("Wait Until Done")) -> (reference out=w670:refnum<vi>, error out=w661:errorcluster)  [unwired: 2 in, 3 out]
      }
      event Value Change {
        w686 = FALSE ("Wait Until Done")
        n261 = event-data() -> ()  [unwired: 1 in, 6 out]
        n262 = invoke class="VI" method="Abort VI"(reference=w680) -> (error out=w679:errorcluster)  [unwired: 2 in, 2 out]
        n263 = call <vilib>:"Clear Errors.vi"("error in (no error)"=w679) -> ("error out"=w678:errorcluster)  [unwired: 5 in, 1 out]
        n264 = flat-sequence {
          tunnel: w678 -> [w694]
          tunnel: [w694] -> w675
          frame #0 {
            n265 = call "stable settings.vi"() -> ()  [unwired: 1 in]
          }
        }
        n266 = case shown="\"measure stable current\"" "Stable Data" {
          tunnel: [w690 w691 w692 w693] -> w677
          frame "measure stable current with transmission" {
            n267 = vi-ref "measure stable current with transmission.vi"() -> (w690:refnum<vi>)
          }
          frame "measure stable current" {
            n268 = vi-ref "measure stable current.vi"() -> (w691:refnum<vi>)
          }
          frame "35Cl + 37Cl measure stable current" {
            n269 = vi-ref "35Cl + 37Cl inj - 35Cl HE.vi"() -> (w692:refnum<vi>)
          }
          frame "35Cl + 37Cl inj - 35Cl HE" {
            n270 = vi-ref "35Cl + 37Cl inj - 35Cl HE.vi"() -> (w693:refnum<vi>)
          }
        }
        n271 = invoke class="VI" method="Run VI"(reference=w677, error in=w675, "Wait until done"=w686, "Auto Dispose Ref"=w686) -> (reference out=w672:refnum<vi>, error out=w687:errorcluster)  [unwired: 1 in, 3 out]
        n272 = invoke on="stable data display" class="SubPnl" method="Insert VI"(error in=w687, "VI Ref"=w672) -> (error out=w673:errorcluster)  [unwired: 2 in, 3 out]
      }
    }
    "Event structure error out" <- w49
    "stable data out" <- w45
    "millisecond timer value" <- w27
    "data" <- w40
    "Measurement values 2" <- w28
    "Sample information" <- w37
    "Measurement values 3" <- w28
    "DAQ state control" <- w30
    n273 = Equal?(x=main_state_control."wait", y=w30) -> (x = y?=w35:bool)
    n274 = shared-variable "My Computer\\DAQuiri shared var.lvlib\\DAQ running"(w35) -> (error out=→"DAQ running SV error":errorcluster)  [unwired: 1 in]
  }
